vi "Main.vi"() -> ()   [LabVIEW 2019]
doc: "This template is for the Queued Message Handler design pattern.\n\nThe Event Handling Loop generates messages based on user interface actions.\n\nThe Message Handling Loop processes messages generated by the Event Handling Loop, or by other messages. The messages are string values, so new messages can be added easily to the Message Cases case structure in the Message Handling Loop. Each message cluster can also provide an optional value for Message Data, which is a variant that can be converted to whatever message-specific data is required."
uses:
  Type_Def/Onglet.ctl
  <vilib>/MakerHub/PS4-Controller/Private/Type Defs/Indicators/Controller.ctl
  <vilib>/MakerHub/PS4-Controller/Private/Type Defs/Indicators/Square.ctl
  <vilib>/MakerHub/PS4-Controller/Private/Type Defs/Indicators/X.ctl
  <vilib>/MakerHub/PS4-Controller/Private/Type Defs/Indicators/Circle.ctl
  <vilib>/MakerHub/PS4-Controller/Private/Type Defs/Indicators/Triangle.ctl
  <vilib>/MakerHub/PS4-Controller/Private/Type Defs/Indicators/L1.ctl
  <vilib>/MakerHub/PS4-Controller/Private/Type Defs/Indicators/R1.ctl
  <vilib>/MakerHub/PS4-Controller/Private/Type Defs/Indicators/Share.ctl
  <vilib>/MakerHub/PS4-Controller/Private/Type Defs/Indicators/Options.ctl
  <vilib>/MakerHub/PS4-Controller/Private/Type Defs/Indicators/PS.ctl
  <vilib>/MakerHub/PS4-Controller/Private/Type Defs/Indicators/Pad_Button.ctl
  <vilib>/MakerHub/PS4-Controller/Private/Type Defs/Indicators/Dpad.ctl
  <vilib>/MakerHub/PS4-Controller/Private/Type Defs/Indicators/Slider.ctl
  <vilib>/MakerHub/PS4-Controller/Private/Type Defs/Buttons.ctl
  <vilib>/MakerHub/PS4-Controller/Private/Type Defs/Axis.ctl
  <vilib>/MakerHub/PS4-Controller/Private/Type Defs/Indicators/DPad Enum.ctl
  Sous-Vi/SSH/SSH Library/Connection Info..cluster.ctl
  Sous-Vi/SSH/SSH Library/Password..cluster.ctl
  Sous-Vi/SSH/SSH Library/Private Public Key..cluster.ctl
  controls/UI Data.ctl
  Type_Def/Data.ctl
  Sous-Vi/SSH/SSH Library/connect_password.vi
  Sous-Vi/SSH/SSH Library/connect_key.vi
  support/Message Queue/Enqueue Message (Single).vi
  <vilib>/Utility/error.llb/Error Cluster From Error Code.vi
  <vilib>/Instr/_visa.llb/VISA Configure Serial Port (Instr).vi
  <vilib>/MakerHub/PS4-Controller/Public/Open First Controller.vi
  <vilib>/Utility/inputDevices.llb/closeJoystick.vi
  <vilib>/Utility/inputDevices.llb/joystickAcquire.vi
  Global/Global_1.vi
  <vilib>/ErrorRing/Error Ring.xnode
  support/Message Queue/Message Queue.lvlib
  support/User Event - Stop/User Event - Stop.lvlib
  <vilib>/MakerHub/PS4-Controller/LMH-PS4.lvlib
  Sous-Vi/SSH/SSH Library/LabSSH.lvlib
panel:
  out "OTHER 2":bool
  in  "Vitesse (ms)":u32(slide)=400 step=100 scale=600.0..100.0
  out "StatCom 2":bool
  in  "Putty":bool
  in  "Stop_Hexap":bool
  in  "Start_Hexap":bool
  in  "Stop COM":bool
  in  "Start COM":bool
  out "StatControll":bool
  out "StatCom":bool
  in  "Home Button":bool
  in  "Preferences Button":bool
  in  "Tab Control":T1
  in  "External_C":enum32{"PS4", "OTHER"}(tab)
  out "PS4 Controller":T2={"Square Button"=FALSE, "X Button"=FALSE, "Circle Button"=FALSE, "Triangle Button"=FALSE, "L1"=FALSE, "R1"=FALSE, "Share Button"=FALSE, "Options Button"=FALSE, "PS Button"=FALSE, "Pad Button"=FALSE, "D-Pad"=5, "L2"=0, "R2"=0, "Thumbstick_Left"={[], []}, "Thumbstick_Right"={[], []}} {"R2" scale=-32768.0..32767.0; "L2" scale=-32768.0..32767.0}
  out "PS4 Buttons":T15
  out "PS4 All Axis":T16
  out "axis info":T18
  out "button":T19
  out "direction info":T20
  out "Nuber of joysticks found:":i32
  in  "Joystick Number":i32
  out "Joystick in Use":T21={"axes total"=6, "buttons total"=14, "pov total"=1, "device name"="Wireless Controller"}
  out "Txt Display":string
  out "button 10":bool
  out "button 9":bool
  out "button 8":bool
  out "button 6":bool
  out "button 7":bool
  out "button 5":bool
  out "button 4":bool
  out "button 3":bool
  out "button 2":bool
  out "button 1":bool
  in  "Type External":enum16{"PS4 commander", "Other"}(ring)
  in  "Button 2":T22
  in  "Right joystick Horizontal 2":u8(slide) scale=3.0..253.0
  in  "Right  joystick Vertical 2":u8(slide) scale=3.0..253.0
  in  "Left joystick Horizontal 2":u8(slide) scale=3.0..253.0
  in  "Left joystick Vertical 2":u8(slide) scale=3.0..253.0
  out "Chaîne":string
  in  "TCP":T23={"port"=8888, "adresse"="", "timeout ms"=1000, "connection ID"=refnum}
  in  "Send":bool
  out "Array 2":u8[](array[numeric]) format="%x"
  out "Array":u8[](array[numeric]) format="%x"
  in  "R/W":bool
  in  "USB":T24={"COM"="", "baud rate (9600)"=34800, "data bits (8)"=8, "parity (0:none)"=enum."None", "stop bits (10: 1 bit)"=10, "flow control (0:none)"=0, "timeout (10sec)"=100} {"stop bits (10: 1 bit)" items=["1.0"=10, "1.5"=15, "2.0"=20]; "flow control (0:none)" items=["None", "XON/XOFF", "RTS/CTS", "XON/XOFF & RTS/CTS", "DTR/DSR", "XON/XOFF & DTR/DSR"]}
  in  "Send_L":bool
  in  "SSH_Connect":bool
  out "Method Response":string
  out "Connected":bool
  in  "Commande":string
  out "Output":string
  in  "Expected Response":string
  in  "Connection Type":enum16{"Password", "Private Key"}(ring)
  in  "Connection Name":string="ERAA_HEXAP"
  in  "Private_Public Key":T25
  in  "Password":T26={"Password"="edison"}
  in  "Connection Info.":T27={"Remote"="192.168.43.226", "Username"="root", "Port (22)"=22}
  out "error_":errorcluster
  out "Chaîne_CONTROLLER":string
  out "Chaîne_USB/WIFI":string
  out "error_Read_Com_SSH":errorcluster
  out "error_Send_Com_SSH":errorcluster
  out "Hexap_ON":bool
  out "Start/Stop COM":bool
  out "USB/WIFI":bool
  out "COM_OK":bool
  out "Init_Controller_OK":bool
  out "Init_COM_OK":bool
  out "Button":T22
  out "Right joystick Horizontal":u8(slide) scale=3.0..253.0
  out "Right  joystick Vertical":u8(slide) scale=3.0..253.0
  out "Left joystick Horizontal":u8(slide) scale=3.0..253.0
  out "Left joystick Vertical":u8(slide) scale=3.0..253.0
  out "Controller_OK":bool
  out "Tab_Ref":refnum<vi>[](array[refnum])
  out "error_OpenUSB":errorcluster
  out "CONTROLER":bool
  out "OTHER":bool
  out "error_Controller":errorcluster
  out "error_Send_Data":errorcluster
  out "error_OpenManette 2":errorcluster
  in  "Search Button":bool
  in  "Settings Button":bool
  in  "Type Comm":T28(ring)
  in  "Type Connexion":enum16{"Connexion USB", "Connexion WIFI"}(ring)=enum."Connexion WIFI"
  # "Debeugue SSH Selement en Exe"
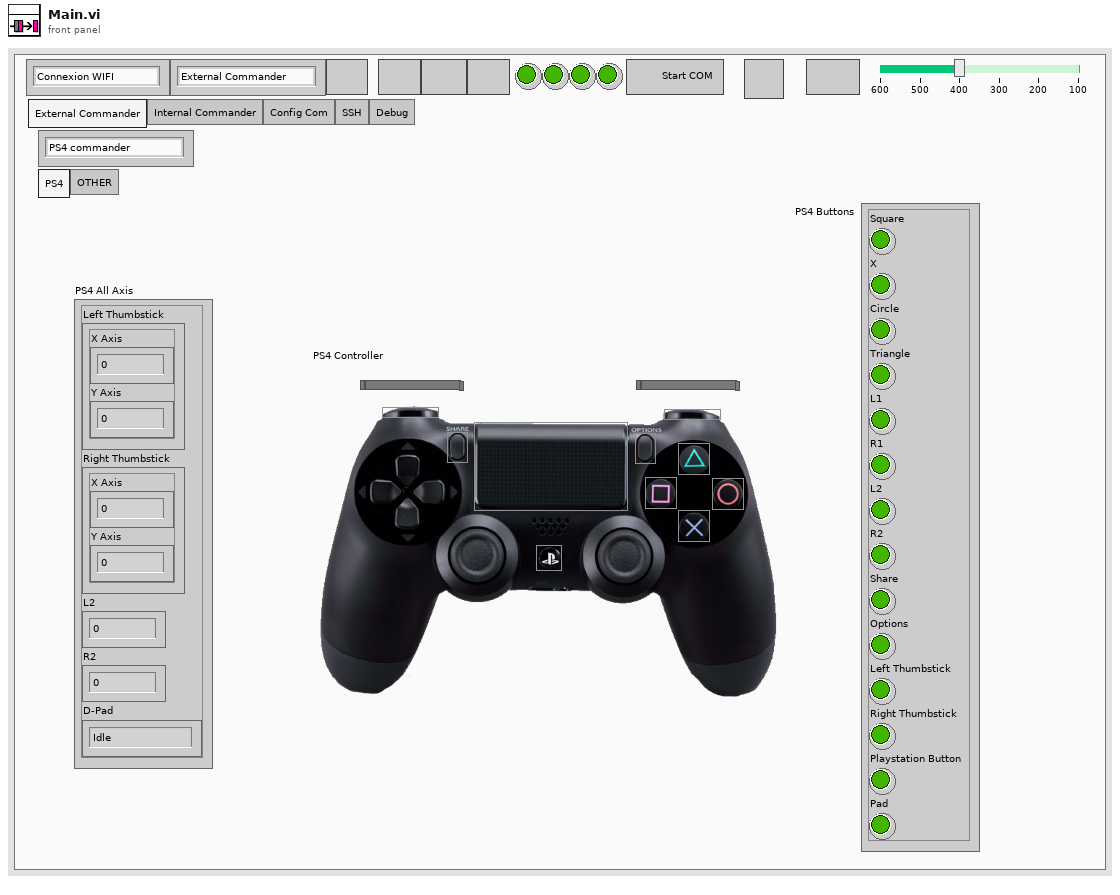
[diagram p1: front panel]
types:
  T1 = typedef "Onglet.ctl" = enum32{"External Commander", "Internal Commander", "Config Com", "SSH", "Debug"}
  T2 = typedef "LMH-PS4.lvlib/Controller.ctl" = cluster{"Square Button":T3, "X Button":T4, "Circle Button":T5, "Triangle Button":T6, "L1":T7, "R1":T8, "Share Button":T9, "Options Button":T10, "PS Button":T11, "Pad Button":T12, "D-Pad":T13, "L2":T14, "R2":T14, "Thumbstick_Left":cluster{i32[], i32[]}, "Thumbstick_Right":cluster{i32[], i32[]}}
  T3 = typedef "LMH-PS4.lvlib/Square.ctl" = bool
  T4 = typedef "LMH-PS4.lvlib/X.ctl" = bool
  T5 = typedef "LMH-PS4.lvlib/Circle.ctl" = bool
  T6 = typedef "LMH-PS4.lvlib/Triangle.ctl" = bool
  T7 = typedef "LMH-PS4.lvlib/L1.ctl" = bool
  T8 = typedef "LMH-PS4.lvlib/R1.ctl" = bool
  T9 = typedef "LMH-PS4.lvlib/Share.ctl" = bool
  T10 = typedef "LMH-PS4.lvlib/Options.ctl" = bool
  T11 = typedef "LMH-PS4.lvlib/PS.ctl" = bool
  T12 = typedef "LMH-PS4.lvlib/Pad_Button.ctl" = bool
  T13 = typedef "LMH-PS4.lvlib/Dpad.ctl" = u16
  T14 = typedef "LMH-PS4.lvlib/Slider.ctl" = i32
  T15 = typedef "LMH-PS4.lvlib/Buttons.ctl" = cluster{"Square":bool, "X":bool, "Circle":bool, "Triangle":bool, "L1":bool, "R1":bool, "L2":bool, "R2":bool, "Share":bool, "Options":bool, "Left Thumbstick":bool, "Right Thumbstick":bool, "Playstation Button":bool, "Pad":bool}
  T16 = typedef "LMH-PS4.lvlib/Axis.ctl" = cluster{"Left Thumbstick":cluster{"X Axis":i32, "Y Axis":i32}, "Right Thumbstick":cluster{"X Axis":i32, "Y Axis":i32}, "L2":i32, "R2":i32, "D-Pad":T17}
  T17 = typedef "LMH-PS4.lvlib/DPad Enum.ctl" = enum16{"Idle", "Up", "Up / Right", "Right", "Down / Right", "Down", "Down / Left", "Left", "Up / Left"}
  T18 = cluster{"X axis":i32, "Y axis":i32, "Z axis":i32, "X axis rotation":i32, "Y axis rotation":i32, "Z axis rotation":i32, "U axis":i32, "V axis":i32}
  T19 = cluster{"button[1]":bool, "button[2]":bool, "button[3]":bool, "button[4]":bool, "button[5]":bool, "button[6]":bool, "button[7]":bool, "button[8]":bool, "button[9]":bool, "button[10]":bool}
  T20 = cluster{"pov 1":i32, "pov 2":i32, "pov 3":i32, "pov 4":i32}
  T21 = cluster{"axes total":u32, "buttons total":u32, "pov total":u32, "device name":string}
  T22 = cluster{"R1":bool, "R2":bool, "R3":bool, "L4":bool, "L5":bool, "L6":bool, "LT":bool, "RT":bool}
  T23 = cluster{"port":u16, "adresse":string, "timeout ms":i32, "connection ID":refnum<k5>}
  T24 = cluster{"COM":refnum<visa-resource-name>, "baud rate (9600)":u32, "data bits (8)":u16, "parity (0:none)":enum16{"None", "Odd", "Even", "Mark", "Space"}, "stop bits (10: 1 bit)":u16, "flow control (0:none)":u16, "timeout (10sec)":u32}
  T25 = typedef "LabSSH.lvlib/Private Public Key..cluster.ctl" = cluster{"Private Key":path, "Passphrase":string}
  T26 = typedef "LabSSH.lvlib/Password..cluster.ctl" = cluster{"Password":string}
  T27 = typedef "LabSSH.lvlib/Connection Info..cluster.ctl" = cluster{"Remote":string, "Username":string, "Port (22)":i32}
  T28 = enum16{"External Commander", "Internal Commander"}
  T29 = typedef "UI Data.ctl" = cluster{"Boolean <Replace Me>":bool, "String <Replace Me>":string, "Numeric <Replace Me>":dbl, "Do Something Ref":refnum<vi>, "Do Something Else Ref":refnum<vi>, "Data Display Ref":refnum<vi>, "Exit Button Ref":refnum<vi>}
  T30 = typedef "Message Queue.lvlib/All Message Queues.ctl" = cluster{"UI":refnum<queue>, "UI 2":refnum<queue>, "UI 3":refnum<queue>, "UI 4":refnum<queue>}
  T31 = typedef "Data.ctl" = cluster{"Data":string, "COM":refnum<visa-resource-name>}
  T32 = typedef "LMH-PS4.lvlib/PS4 Controller Ref.ctl" = cluster{"Controller Ref":refnum<k1>, "PS4 Events Ref":refnum<event-registration>, "Worker Ref":refnum<vi>}
  T33 = cluster{"axes total":u32, "buttons total":u32, "pov total":u32, "device name":string}[]
  T34 = cluster{"button 1":bool, "button 2":bool, "button 3":bool, "button 4":bool, "button 5":bool, "button 6":bool, "button 7":bool, "button 8":bool, "button 9":bool, "button 10":bool, "button 11":bool, "button 12":bool, "button 13":bool, "button 14":bool, "button 15":bool, "button 16":bool, "button 17":bool, "button 18":bool, "button 19":bool, "button 20":bool, "button 21":bool, "button 22":bool, "button 23":bool, "button 24":bool, "button 25":bool, "button 26":bool, "button 27":bool, "button 28":bool, "button 29":bool, "button 30":bool, "button 31":bool, "button 32":bool}
  T35 = cluster{"button info[0]":bool, "button info[1]":bool, "button info[2]":bool, "button info[3]":bool, "button info[4]":bool, "button info[5]":bool, "button info[6]":bool, "button info[7]":bool, "button info[8]":bool, "button info[9]":bool}
  T36 = cluster{"Boolean array[0]":bool, "Boolean array[1]":bool, "Boolean array[2]":bool, "Boolean array[3]":bool, "Boolean array[4]":bool, "Boolean array[5]":bool, "Boolean array[6]":bool, "Boolean array[7]":bool, "Boolean array[8]":bool}
  T37 = enum32{"External Commander", "Internal Commander", "Config Com", "SSH", "Debug"}
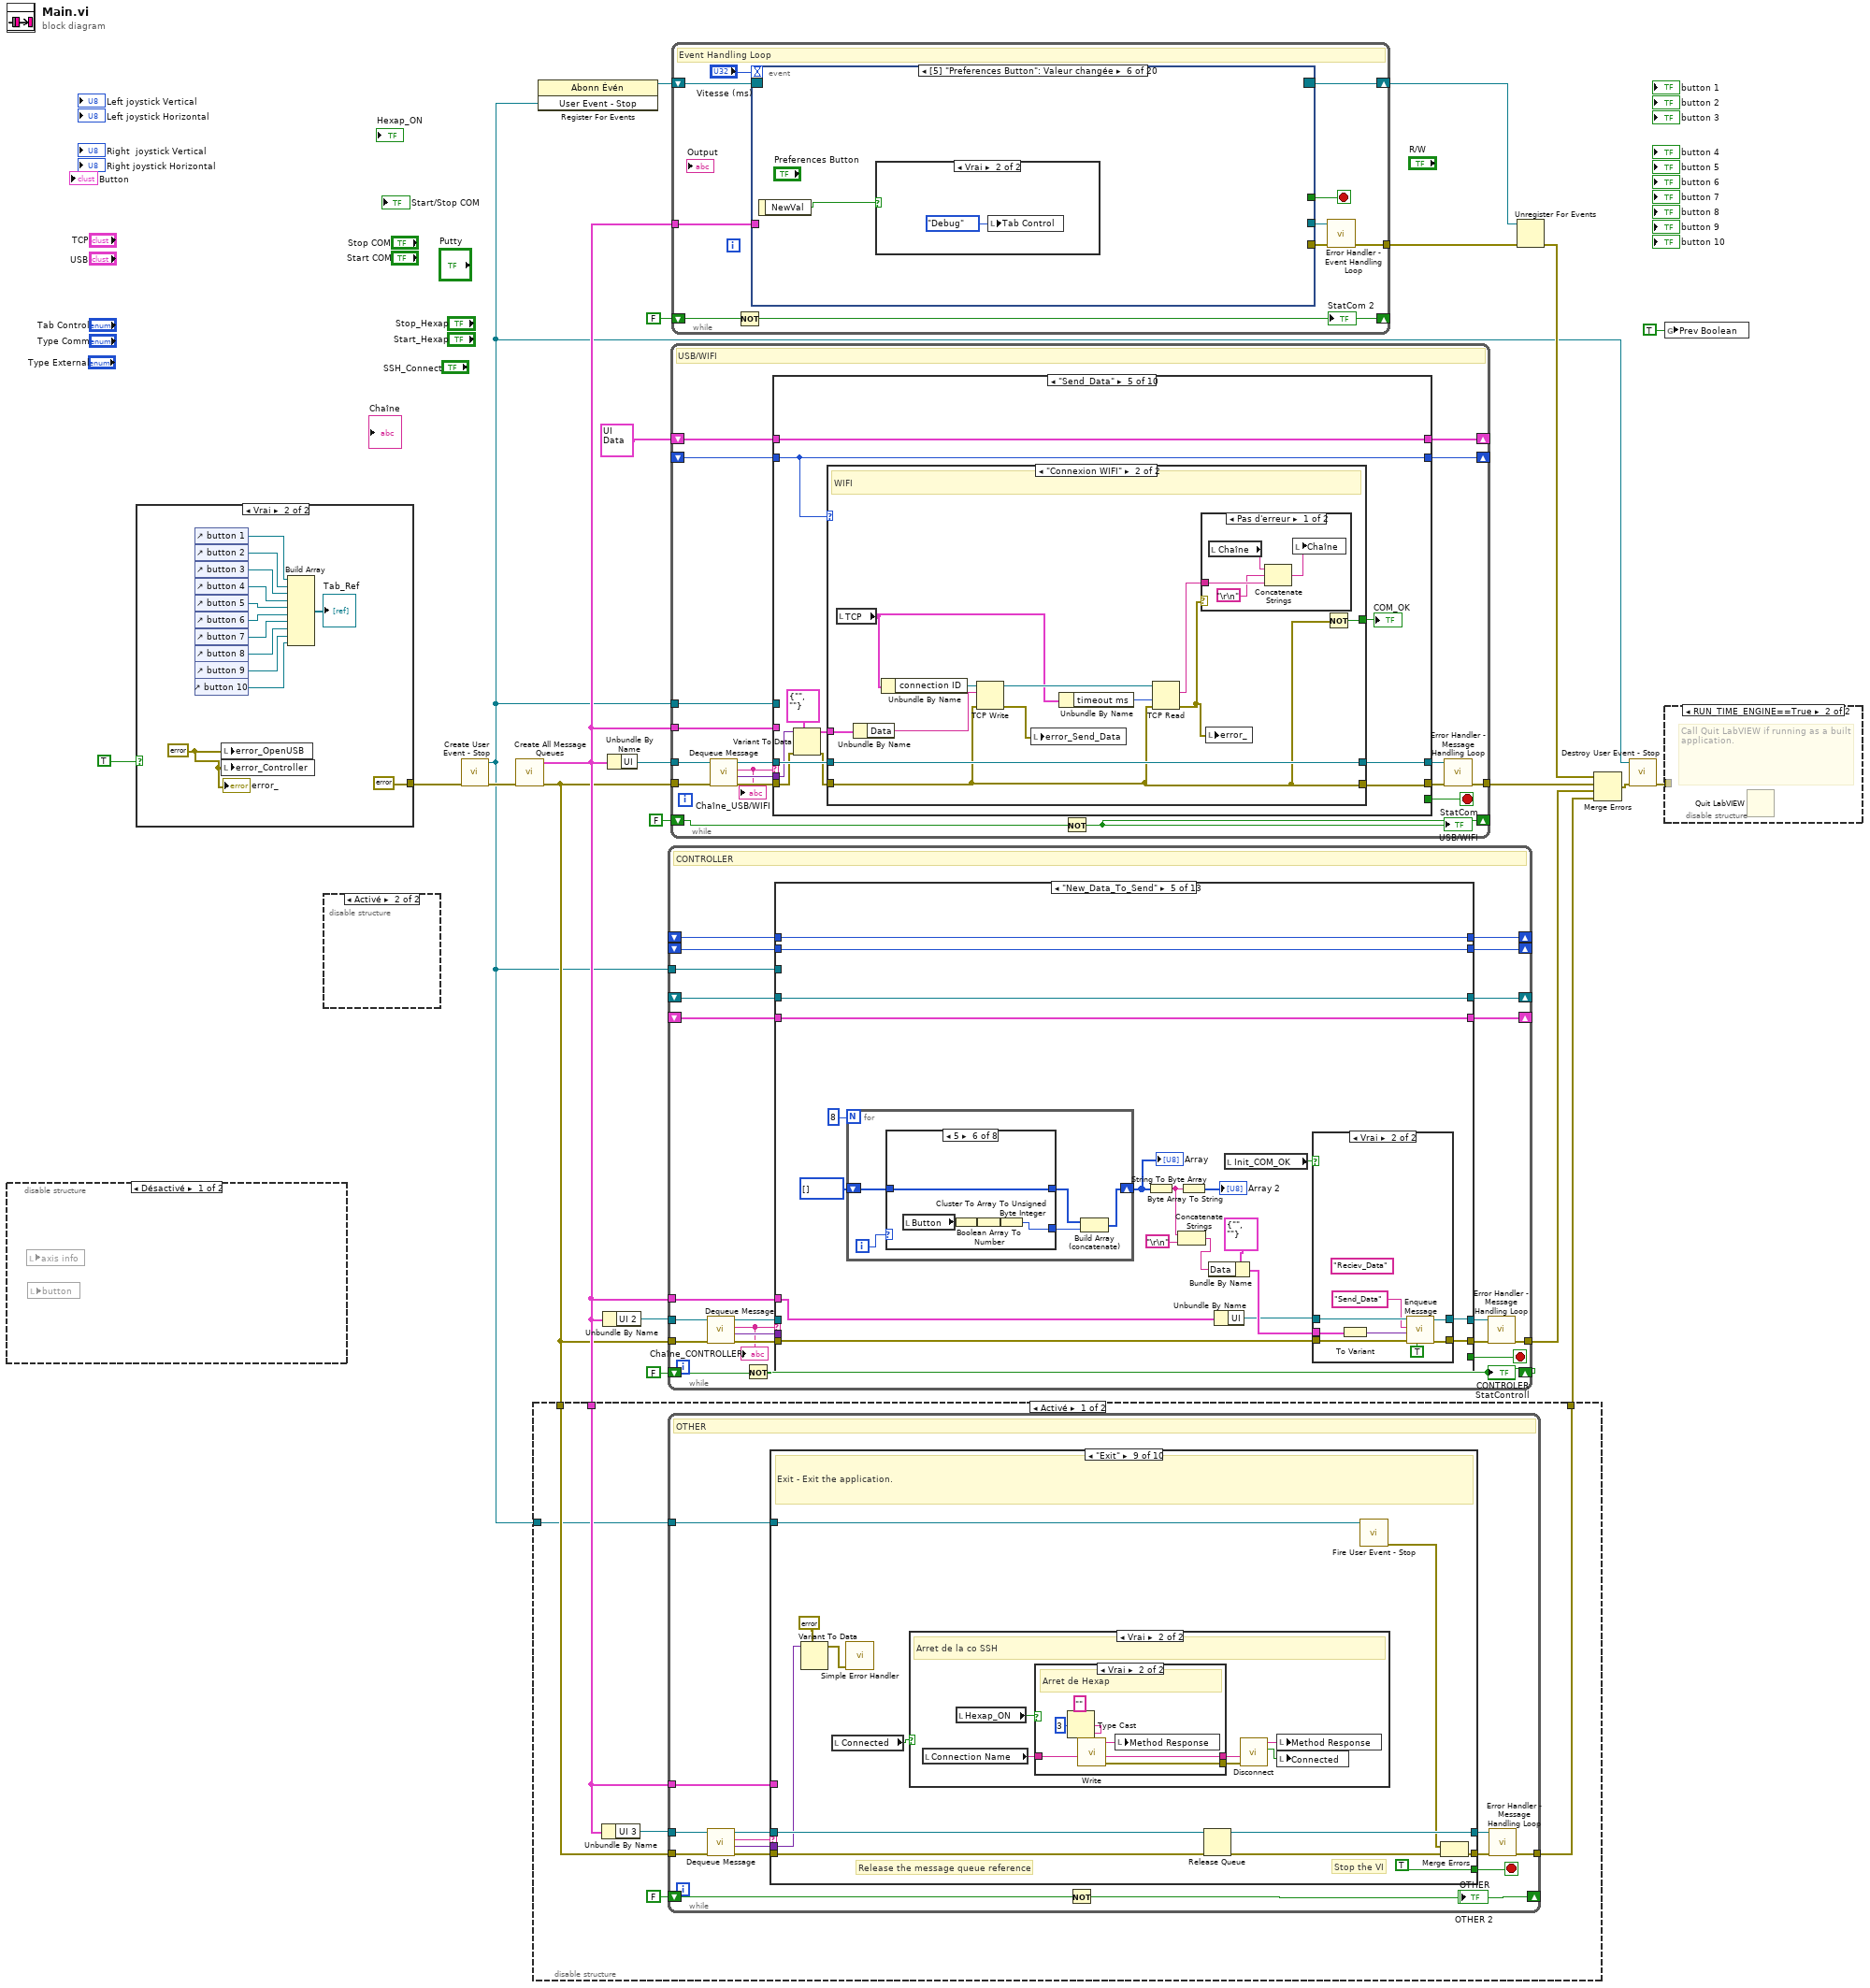
[diagram p0: block diagram]
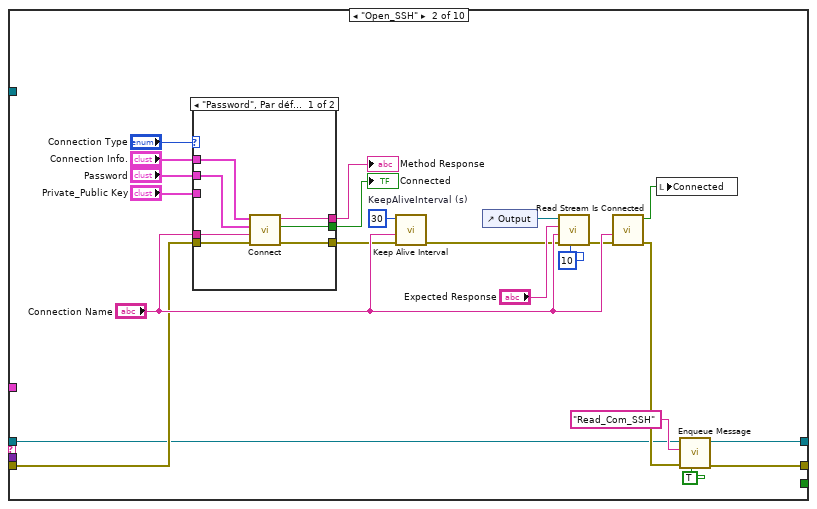
[diagram p4: hidden frame]
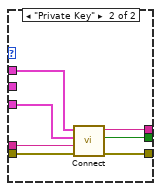
[diagram p5: hidden frame]
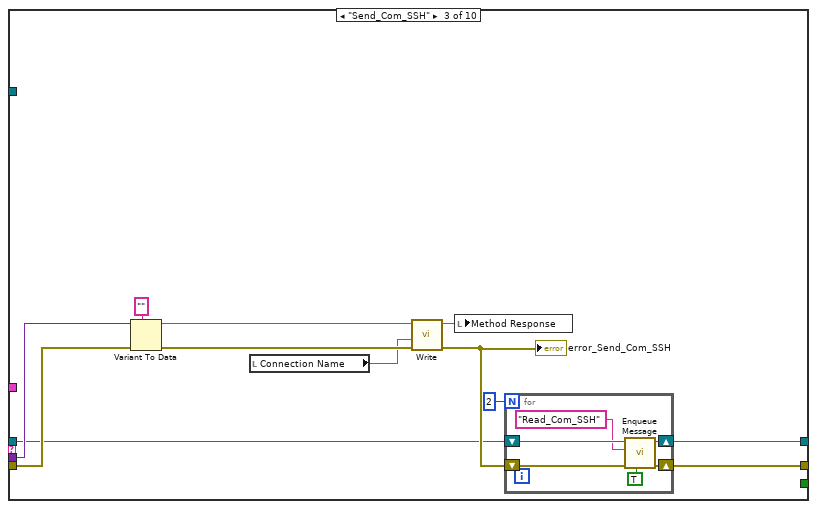
[diagram p6: hidden frame]
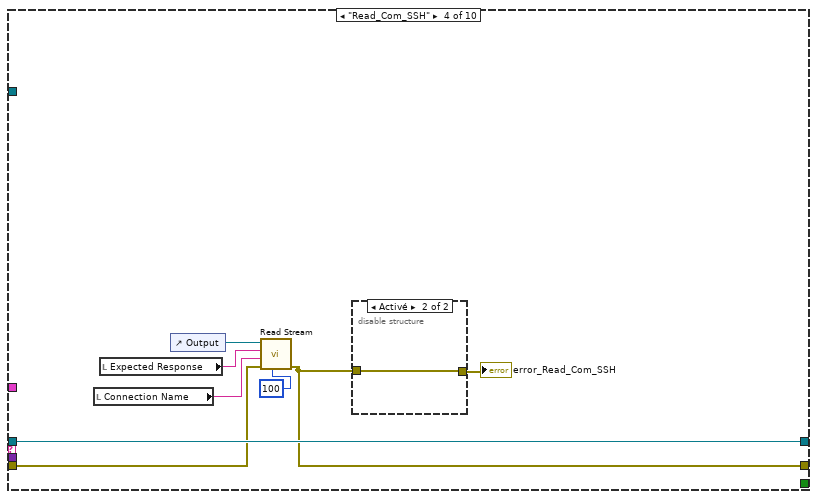
[diagram p7: hidden frame]
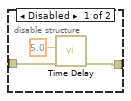
[diagram p8: hidden frame]
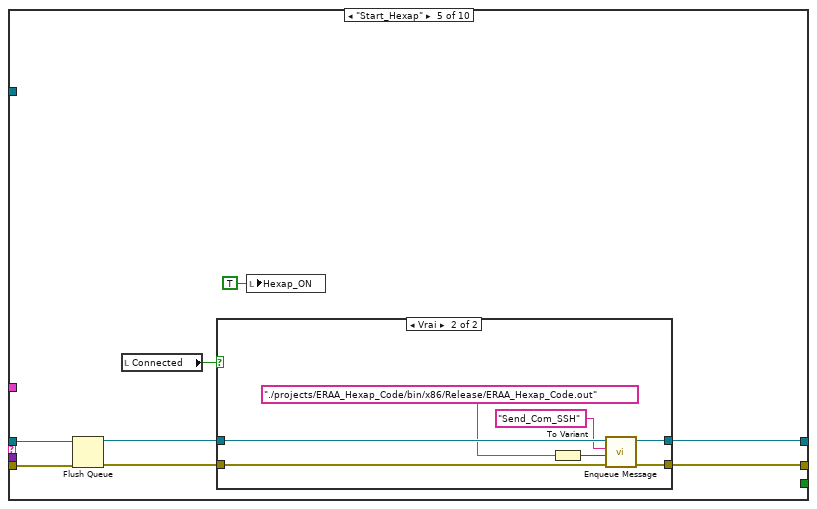
[diagram p9: hidden frame]
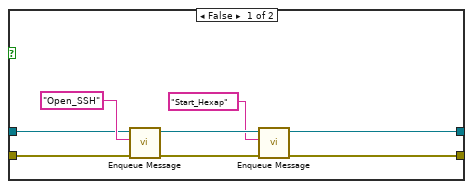
[diagram p10: hidden frame]
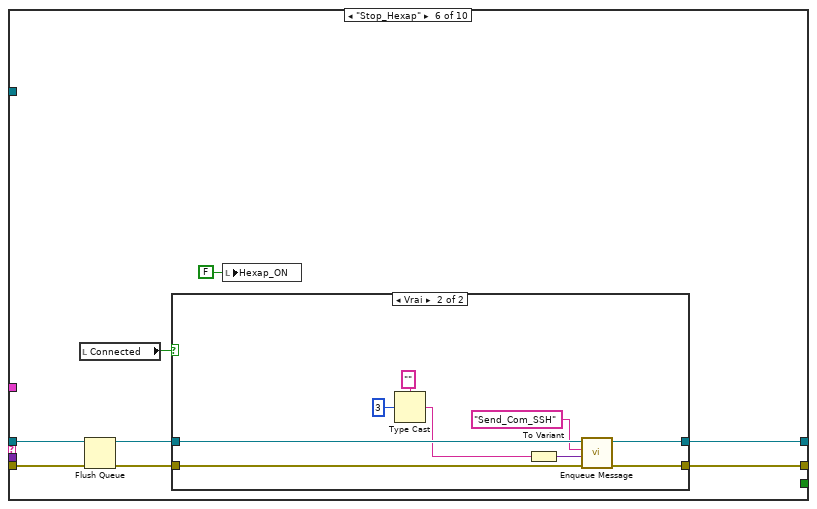
[diagram p11: hidden frame]
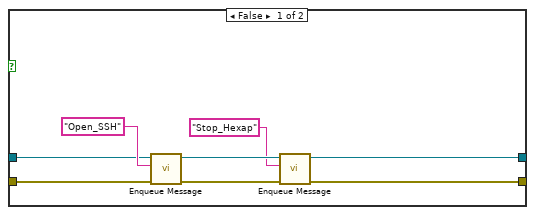
[diagram p12: hidden frame]
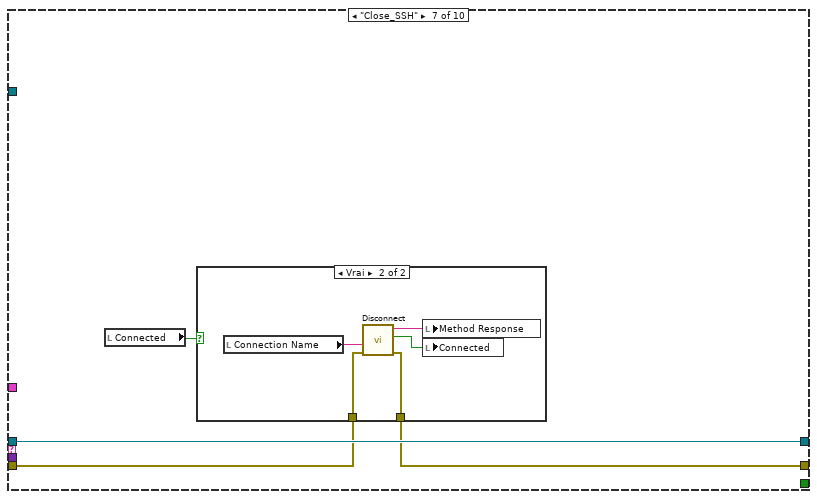
[diagram p13: hidden frame]
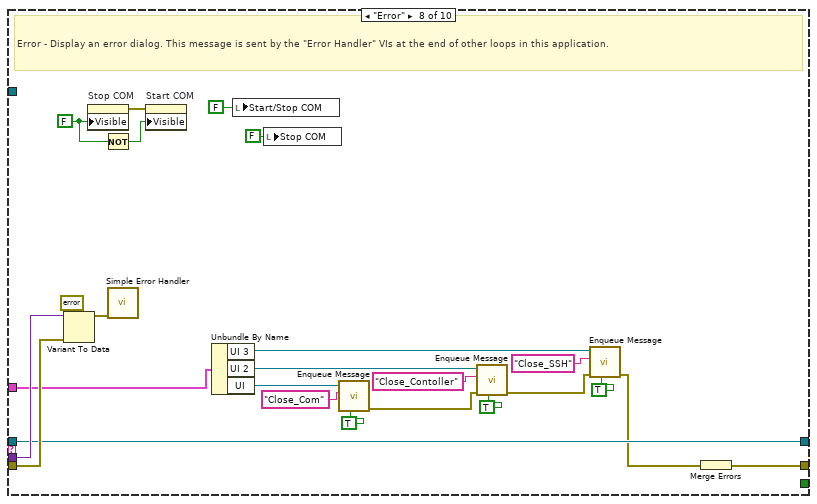
[diagram p15: hidden frame]
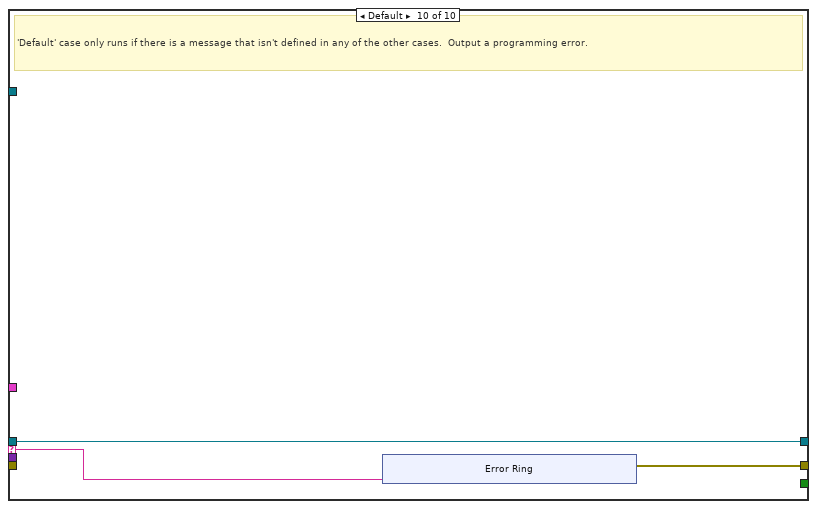
[diagram p18: hidden frame]
diagram:
  n1 = disable-structure shown="Désactivé" {
    frame Disabled {
      n2 = local read "axis info"() -> ()  [unwired: 1 in]
      n3 = local read "button"() -> ()  [unwired: 1 in]
    }
    frame Enabled {
    }
  }
  n4 = case shown="Vrai" TRUE {
    tunnel: [_ errorcluster {"status"=FALSE, "code"=0, "source"=""} ("error out")] -> w7
    frame False {
    }
    frame True {
      w23 = errorcluster {"status"=FALSE, "code"=0, "source"=""} ("error out")
      n5 = control-ref of="button 1"() -> (w25:refnum<vi>)
      n6 = control-ref of="button 2"() -> (w26:refnum<vi>)
      n7 = control-ref of="button 3"() -> (w27:refnum<vi>)
      n8 = control-ref of="button 4"() -> (w28:refnum<vi>)
      n9 = control-ref of="button 5"() -> (w29:refnum<vi>)
      n10 = control-ref of="button 6"() -> (w30:refnum<vi>)
      n11 = control-ref of="button 7"() -> (w31:refnum<vi>)
      n12 = control-ref of="button 8"() -> (w32:refnum<vi>)
      n13 = control-ref of="button 9"() -> (w33:refnum<vi>)
      n14 = control-ref of="button 10"() -> (w34:refnum<vi>)
      n15 = local write "error_OpenUSB"(w23) -> ()
      n16 = local write "error_Controller"(w23) -> ()
      n17 = Build Array(w25, w26, w27, w28, w29, w30, w31, w32, w33, w34) -> (→"Tab_Ref":refnum<vi>[])
      "error_" <- w23
    }
  }
  n18 = disable-structure shown="Activé" {
    frame Disabled {
      n19 = call <vilib>:"Disconnect Network Resource.vi"() -> ()  [unwired: 7 in, 1 out]
      n20 = call <vilib>:"Add Network Resource.vi"() -> ()  [unwired: 7 in, 1 out]
      n21 = global read "Global_1.vi" item#-1() -> ()  [unwired: 1 in]
    }
    frame Enabled {
    }
  }
  n22 = call "Create User Event - Stop.vi"("error in (no error)"=w7) -> ("error out"=w20:errorcluster, "User Event - Stop"=w1:refnum<user-event>)  [unwired: 9 in]
  n23 = call "Create All Message Queues.vi"("error in (no error)"=w20) -> ("error out"=w4:errorcluster, "Message Queues out"=w10:T30)  [unwired: 9 in]
  n24 = disable-structure shown="Activé" {
    disable-tunnel: w10 -> [w37 _]
    disable-tunnel: [w40 w240] -> w9
    disable-tunnel: w4 -> [w38 w240]
    disable-tunnel: w1 -> [w36 _]
    frame Enabled {
      n25 = Unbundle By Name(w37) -> ("UI 3"=w41:refnum<queue>)
      n26 = while {
        tunnel: w41 -> [w51]
        shift-right: [w42] -> _
        shift-left: FALSE -> [w46]
        tunnel: w38 -> [w45]
        tunnel: [w49] -> w40
        tunnel: w37 -> [w44]
        tunnel: w36 -> [w43]
        stop <- w55 stop-if-true
        # "OTHER"
        n27 = call "Dequeue Message.vi"("error in (no error)"=w45, "Message Queue"=w51) -> ("error out"=w54:errorcluster, "Message Data"=w52:variant, "Message"=w53:string, "dup Message Queue"=w50:refnum<queue>)  [unwired: 6 in]
        n28 = case "Message Cases" shown="\"Exit\"" w53 {
          selector: w53 -> [_ _ _ _ _ _ _ _ _ w231]
          tunnel: w50 -> [w57 w60 w96 w119 w127 w148 w175 w200 w216 w230]
          tunnel: w54 -> [w56 w61 w97 w113 w126 w147 w173 w205 w212 _]
          tunnel: [w56 w58 w94 w112 w124 w149 w172 w201 w213 w232] -> w48
          tunnel: [_ _ _ _ _ _ _ _ TRUE _] -> w55
          tunnel: w52 -> [_ _ w98 _ _ _ _ w204 w209 _]
          tunnel: [w57 w59 w95 w119 w125 w150 w175 w200 w216 w230] -> w47
          tunnel: w44 -> [_ _ _ _ _ _ _ w188 _ _]
          tunnel: w43 -> [_ _ _ _ _ _ _ _ w206 _]
          frame "Initialize" {
            # "Initialize - All initialization work should take place in this message, since other loops can potentially enqueue messages that execute immediately after this one."
          }
          frame "Open_SSH" {
            w62 = 30  # KeepAliveInterval (s)
            n29 = case shown="\"Password\", Par défaut" "Connection Type" {
              tunnel: "Connection Info." -> [w86 w91]
              tunnel: "Password" -> [w85 _]
              tunnel: "Private_Public Key" -> [_ w90]
              tunnel: w61 -> [w84 w93]
              tunnel: [w83 w92] -> w72
              tunnel: "Connection Name" -> [w82 w89]
              tunnel: [w81 w88] -> w71
              tunnel: [w80 w87] -> w70
              frame "Password", Default {
                n30 = call-poly "Connect.vi"("error in (no error)"=w84, "Connection Name"=w82, "Password"=w85, "Connection Info."=w86) -> ("error out"=w83:errorcluster, "isSshConnected"=w80:bool, "Return String"=w81:string)  [unwired: 5 in]
              }
              frame "Private Key" {
                n31 = call-poly "Connect.vi"("error in (no error)"=w93, "Connection Name"=w89, "Private_Public Key"=w90, "Connection Info."=w91) -> ("error out"=w92:errorcluster, "isSshConnected"=w87:bool, "Return String"=w88:string)  [unwired: 5 in]
              }
            }
            "Connected" <- w70
            "Method Response" <- w71
            n32 = call "Keep Alive Interval.vi"("error in (no error)"=w72, "Connection Name"="Connection Name", "KeepAliveInterval (s)"=w62) -> ("error out"=w74:errorcluster)  [unwired: 8 in]
            n33 = control-ref of="Output"() -> (w73:refnum<vi>)
            n34 = call "Read Stream.vi"("Timout (ms)"=10 ("Timout (s)"), "error in (no error)"=w74, "Connection Name"="Connection Name", "Expected Response"="Expected Response", "Output ref"=w73) -> ("error out"=w76:errorcluster)  [unwired: 6 in]
            n35 = call "Is Connected.vi"("error in (no error)"=w76, "Connection Name"="Connection Name") -> ("error out"=w79:errorcluster, "isSshConnected"=w78:bool)  [unwired: 8 in]
            n36 = local write "Connected"(w78) -> ()
            n37 = call-poly "Enqueue Message.vi"("Priority Message? (F)"=TRUE, "error in (no error)"=w79, "Message"="Read_Com_SSH", "Message Queue"=w60) -> ("error out"=w58:errorcluster, "dup Message Queue"=w59:refnum<queue>)  [unwired: 6 in]
          }
          frame "Send_Com_SSH" {
            n38 = Variant To Data(error in=w97, type="" ("Commande"), Variant=w98) -> (data=w104:string, error out=w102:errorcluster)
            n39 = local read "Connection Name"() -> (w101:string)
            n40 = call "Write.vi"("error in (no error)"=w102, "Connection Name"=w101, "Command"=w104) -> ("error out"=w99:errorcluster, "Return String"=w103:string)  [unwired: 7 in]
            "error_Send_Com_SSH" <- w99
            n41 = local write "Method Response"(w103) -> ()
            n42 = for {
              N: 2 -> [_]
              shift-right: [w109] -> w95
              shift-left: w96 -> [w110]
              shift-right: [w111] -> w94
              shift-left: w99 -> [w107]
              n43 = call-poly "Enqueue Message.vi"("Priority Message? (F)"=TRUE, "error in (no error)"=w107, "Message"="Read_Com_SSH", "Message Queue"=w110) -> ("error out"=w111:errorcluster, "dup Message Queue"=w109:refnum<queue>)  [unwired: 6 in]
            }
          }
          frame "Read_Com_SSH" {
            n44 = local read "Connection Name"() -> (w117:string)
            n45 = local read "Expected Response"() -> (w116:string)
            n46 = control-ref of="Output"() -> (w115:refnum<vi>)
            n47 = call "Read Stream.vi"("Timout (ms)"=100 ("Timout (s)"), "error in (no error)"=w113, "Connection Name"=w117, "Expected Response"=w116, "Output ref"=w115) -> ("error out"=w112:errorcluster)  [unwired: 6 in]
            n48 = disable-structure shown="Activé" {
              disable-tunnel: w112 -> [w121 w123]
              disable-tunnel: [w120 w123] -> w118
              frame Disabled {
                n49 = call "Time Delay"("error in (no error)"=w121, "Delay Time (s)"=5.0) -> ("error out"=w120:errorcluster)  [unwired: 9 in]
              }
              frame Enabled {
              }
            }
            "error_Read_Com_SSH" <- w118
          }
          frame "Start_Hexap" {
            n50 = Flush Queue(queue=w127, error in (no error)=w126) -> (queue out=w130:refnum<queue>, error out=w131:errorcluster)  [unwired: 1 out]
            n51 = local read "Connected"() -> (w129:bool)
            n52 = case shown="Vrai" w129 {
              tunnel: w130 -> [w138 w146]
              tunnel: w131 -> [w137 w145]
              tunnel: [w134 w141] -> w125
              tunnel: [w133 w140] -> w124
              frame False {
                n53 = call-poly "Enqueue Message.vi"("error in (no error)"=w137, "Message"="Open_SSH", "Message Queue"=w138) -> ("error out"=w135:errorcluster, "dup Message Queue"=w136:refnum<queue>)  [unwired: 7 in]
                n54 = call-poly "Enqueue Message.vi"("error in (no error)"=w135, "Message"="Start_Hexap", "Message Queue"=w136) -> ("error out"=w133:errorcluster, "dup Message Queue"=w134:refnum<queue>)  [unwired: 7 in]
              }
              frame True {
                n55 = To Variant(anything="./projects/ERAA_Hexap_Code/bin/x86/Release/ERAA_Hexap_Code.out" ("Message")) -> (Variant=w143:variant)
                n56 = call-poly "Enqueue Message.vi"("error in (no error)"=w145, "Message Data"=w143, "Message"="Send_Com_SSH", "Message Queue"=w146) -> ("error out"=w140:errorcluster, "dup Message Queue"=w141:refnum<queue>)  [unwired: 6 in]
              }
            }
            n57 = local write "Hexap_ON"(TRUE ("Hexap_ON")) -> ()
          }
          frame "Stop_Hexap" {
            n58 = local read "Connected"() -> (w152:bool)
            n59 = Flush Queue(queue=w148, error in (no error)=w147) -> (queue out=w153:refnum<queue>, error out=w154:errorcluster)  [unwired: 1 out]
            n60 = case shown="Vrai" w152 {
              tunnel: w153 -> [w161 w171]
              tunnel: w154 -> [w160 w170]
              tunnel: [w157 w167] -> w150
              tunnel: [w156 w166] -> w149
              frame False {
                n61 = call-poly "Enqueue Message.vi"("error in (no error)"=w160, "Message"="Open_SSH", "Message Queue"=w161) -> ("error out"=w158:errorcluster, "dup Message Queue"=w159:refnum<queue>)  [unwired: 7 in]
                n62 = call-poly "Enqueue Message.vi"("error in (no error)"=w158, "Message"="Stop_Hexap", "Message Queue"=w159) -> ("error out"=w156:errorcluster, "dup Message Queue"=w157:refnum<queue>)  [unwired: 7 in]
              }
              frame True {
                n63 = Type Cast(type="", x=u8 3) -> (*(type *) &x=w163:string)
                n64 = To Variant(anything=w163) -> (Variant=w168:variant)
                n65 = call-poly "Enqueue Message.vi"("error in (no error)"=w170, "Message Data"=w168, "Message"="Send_Com_SSH", "Message Queue"=w171) -> ("error out"=w166:errorcluster, "dup Message Queue"=w167:refnum<queue>)  [unwired: 6 in]
              }
            }
            n66 = local write "Hexap_ON"(FALSE ("Hexap_ON")) -> ()
          }
          frame "Close_SSH" {
            n67 = local read "Connected"() -> (w174:bool)
            n68 = case shown="Vrai" w174 {
              tunnel: w173 -> [w176 w178]
              tunnel: [w176 w177] -> w172
              frame False {
              }
              frame True {
                n69 = local read "Connection Name"() -> (w181:string)
                n70 = call "Disconnect.vi"("error in (no error)"=w178, "Connection Name"=w181) -> ("error out"=w177:errorcluster, "isSshConnected"=w179:bool, "Return String"=w180:string)  [unwired: 7 in]
                n71 = local write "Method Response"(w180) -> ()
                n72 = local write "Connected"(w179) -> ()
              }
            }
          }
          frame "Error" {
            w186 = FALSE
            # "Error - Display an error dialog. This message is sent by the \"Error Handler\" VIs at the end of other loops in this application."
            n73 = Variant To Data(error in=w205, type=errorcluster {"status"=FALSE, "code"=0, "source"=""} ("error constant"), Variant=w204) -> (data=w202:errorcluster)  [unwired: 1 out]
            n74 = property on="Stop COM" class="Bool (strict)"("Visible"=w186) -> (error out=w184:errorcluster)  [unwired: 2 in, 1 out]
            n75 = Not(x=w186) -> (.not. x?=w185:bool)
            n76 = call <vilib>:"Simple Error Handler.vi"("error in (no error)"=w202) -> ()  [unwired: 4 in, 5 out]
            n77 = property on="Start COM" class="Bool (strict)"(error in=w184, "Visible"=w185) -> ()  [unwired: 1 in, 2 out]
            n78 = Unbundle By Name(w188) -> ("UI 3"=w190:refnum<queue>, "UI 2"=w194:refnum<queue>, "UI"=w197:refnum<queue>)
            n79 = local write "Start/Stop COM"(FALSE ("Start/Stop COM")) -> ()
            n80 = local write "Stop COM"(FALSE ("Stop COM")) -> ()
            n81 = call-poly "Enqueue Message.vi"("Priority Message? (F)"=TRUE, "Message"="Close_Com", "Message Queue"=w197) -> ("error out"=w193:errorcluster)  [unwired: 7 in, 1 out]
            n82 = call-poly "Enqueue Message.vi"("Priority Message? (F)"=TRUE, "error in (no error)"=w193, "Message"="Close_Contoller", "Message Queue"=w194) -> ("error out"=w189:errorcluster)  [unwired: 6 in, 1 out]
            n83 = call-poly "Enqueue Message.vi"("Priority Message? (F)"=TRUE, "error in (no error)"=w189, "Message"="Close_SSH", "Message Queue"=w190) -> ("error out"=w187:errorcluster)  [unwired: 6 in, 1 out]
            n84 = Merge Errors(w187) -> (w201:errorcluster)
          }
          frame "Exit" {
            # "Stop the VI"
            # "Release the message queue reference"
            # "Exit - Exit the application."
            n85 = Variant To Data(type=errorcluster {"status"=FALSE, "code"=0, "source"=""} ("error constant"), Variant=w209) -> (data=w210:errorcluster)  [unwired: 1 in, 1 out]
            n86 = local read "Connected"() -> (w208:bool)
            n87 = call <vilib>:"Simple Error Handler.vi"("error in (no error)"=w210) -> ()  [unwired: 4 in, 5 out]
            n88 = case shown="Vrai" w208 {
              frame False {
              }
              frame True {
                # "Arret de la co SSH"
                n89 = local read "Connection Name"() -> (w219:string)
                n90 = local read "Hexap_ON"() -> (w220:bool)
                n91 = case shown="Vrai" w220 {
                  tunnel: w219 -> [w223 w229]
                  tunnel: [w223 w229] -> w218
                  tunnel: [_ w228] -> w217
                  frame False {
                  }
                  frame True {
                    # "Arret de Hexap"
                    n92 = Type Cast(type="", x=u8 3) -> (*(type *) &x=w224:string)
                    n93 = call "Write.vi"("Connection Name"=w229, "Command"=w224) -> ("error out"=w228:errorcluster, "Return String"=w227:string)  [unwired: 8 in]
                    n94 = local write "Method Response"(w227) -> ()
                  }
                }
                n95 = call "Disconnect.vi"("error in (no error)"=w217, "Connection Name"=w218) -> ("isSshConnected"=w221:bool, "Return String"=w222:string)  [unwired: 7 in, 1 out]
                n96 = local write "Method Response"(w222) -> ()
                n97 = local write "Connected"(w221) -> ()
              }
            }
            n98 = Release Queue(queue=w216, error in (no error)=w212) -> (error out=w214:errorcluster)  [unwired: 1 in, 2 out]
            n99 = call "Fire User Event - Stop.vi"("User Event - Stop"=w206) -> ("error out"=w207:errorcluster)  [unwired: 10 in]
            n100 = Merge Errors(w207, w214) -> (w213:errorcluster)
          }
          frame Default {
            # "'Default' case only runs if there is a message that isn't defined in any of the other cases.  Output a programming error."
            n101 = xnode "Error Ring"("paramètre 0"=w231) -> ("sortie d'erreur"=w232:errorcluster)
          }
        }
        n102 = Not(x=w46) -> (.not. x?=w42:bool)
        "OTHER" <- w42
        "OTHER 2" <- w42
        n103 = call "Error Handler - Message Handling Loop.vi"("error in (no error)"=w48, "Message Queue"=w47) -> ("dup error in"=w49:errorcluster)  [unwired: 8 in, 1 out]
      }
    }
    frame Disabled {
    }
  }
  n104 = register-events(w1) -> (reference out=w13:refnum<event-registration>)  [unwired: 2 in, 1 out]
  n105 = Unbundle By Name(w10) -> ("UI 2"=w12:refnum<queue>)
  n106 = Unbundle By Name(w10) -> ("UI"=w21:refnum<queue>)
  n107 = while {
    tunnel: w12 -> [w258]
    tunnel: w4 -> [w261]
    tunnel: [w256] -> w11
    tunnel: w10 -> [w254]
    shift-right: [w252] -> _
    shift-left: _ -> [w251]
    shift-right: [w250] -> _
    shift-left: _ -> [w249]
    shift-right: [w248] -> _
    shift-left: _ -> [w247]
    shift-right: [w246] -> _
    shift-left: _ -> [w245]
    shift-right: [w243] -> _
    shift-left: FALSE -> [w244]
    tunnel: w1 -> [w242]
    stop <- w262 stop-if-true
    # "CONTROLLER"
    n108 = call "Dequeue Message.vi"("error in (no error)"=w261, "Message Queue"=w258) -> ("error out"=w260:errorcluster, "Message Data"=w259:variant, "Message"=w241:string, "dup Message Queue"=w257:refnum<queue>)  [unwired: 6 in]
    "Chaîne_CONTROLLER" <- w241
    n109 = Not(x=w244) -> (.not. x?=w243:bool)
    "CONTROLER" <- w243
    "StatControll" <- w243
    n110 = case "Message Cases" shown="\"New_Data_To_Send\"" w241 {
      selector: w241 -> [_ _ _ _ _ _ _ _ _ _ _ _ w644]
      tunnel: w257 -> [w266 w285 w354 w418 _ _ _ w547 w553 w581 w603 w620 w643]
      tunnel: w260 -> [w265 w284 w359 w419 w488 w529 w539 w548 w557 w586 w599 w619 _]
      tunnel: [w263 errorcluster {"status"=FALSE, "code"=0, "source"=""} ("sortie d'erreur") w355 w422 w486 w527 w537 w548 w558 w582 w600 w618 w645] -> w255
      tunnel: [_ _ _ _ _ _ _ _ _ _ TRUE _ _] -> w262
      tunnel: w259 -> [_ _ _ _ _ _ _ _ w556 w585 w596 _ _]
      tunnel: w254 -> [_ _ _ _ w477 w530 w540 _ _ w560 _ _ _]
      tunnel: [w264 w281 w353 w423 w487 w528 w538 w547 w553 w581 w603 w617 w643] -> w253
      tunnel: [w273 w293 w362 w421 w485 w526 w536 w546 w552 w580 w595 w625 w642] -> w252
      tunnel: w251 -> [w273 _ w362 w421 w485 w526 w536 w546 w552 w580 w595 w625 w642]
      tunnel: [w272 w292 w360 w426 w480 w525 w535 w545 w551 w579 _ _ w641] -> w250
      tunnel: w249 -> [w272 w291 w361 w426 w480 w525 w535 w545 w551 w579 w591 w622 w641]
      tunnel: [w271 w290 w358 w420 w478 w523 w533 w543 w549 w577 w594 w624 w639] -> w248
      tunnel: w247 -> [w271 _ w358 w420 w478 w523 w533 w543 w549 w577 w594 w624 w639]
      tunnel: [w270 w289 w356 w425 w479 w524 w534 w544 w550 w578 _ _ w640] -> w246
      tunnel: w245 -> [w270 w288 w357 w425 w479 w524 w534 w544 w550 w578 w593 w623 w640]
      tunnel: w242 -> [_ _ _ _ _ _ _ _ _ _ w588 _ _]
      frame "Initialize" {
        n111 = local read "Type External"() -> (w267:enum16{"PS4 commander", "Other"})
        n112 = local read "Type Comm"() -> (w268:T28)
        n113 = case shown="\"External Commander\", Par défaut" w268 {
          tunnel: w267 -> [w275 _]
          frame "External Commander", Default {
            n114 = case shown="\"PS4 commander\", Par défaut" w275 {
              frame "PS4 commander", Default {
                n115 = local write "External_C"(enum32{"PS4", "OTHER"}."PS4" ("External_C")) -> ()
              }
              frame "Other" {
                n116 = local write "External_C"(enum32{"PS4", "OTHER"}."OTHER" ("External_C")) -> ()
              }
            }
            n117 = local write "Tab Control"(Onglet."External Commander" ("Tab Control")) -> ()
          }
          frame "Internal Commander" {
            n118 = local write "Tab Control"(Onglet."Internal Commander" ("Tab Control")) -> ()
          }
        }
        n119 = property on="External_C" class="Onglet (strict)"("Tabs Visible?"=FALSE ("Onglets visibles ?")) -> ()  [unwired: 2 in, 2 out]
        n120 = Flush Queue(queue=w266, error in (no error)=w265) -> (queue out=w264:refnum<queue>, error out=w263:errorcluster)  [unwired: 1 out]
      }
      frame "Open_Controller" {
        # "Initialize - All initialization work should take place in this message, since other loops can potentially enqueue messages that execute immediately after this one."
        n121 = local read "Type Comm"() -> (w293:T28)
        n122 = local read "Type External"() -> (w290:enum16{"PS4 commander", "Other"})
        n123 = Flush Queue(queue=w285, error in (no error)=w284) -> (queue out=w282:refnum<queue>, error out=w283:errorcluster)  [unwired: 1 out]
        n124 = case shown="\"External Commander\", Par défaut" w293 {
          tunnel: w282 -> [w303 w350]
          tunnel: w283 -> [w300 w349]
          tunnel: [w303 w350] -> w281
          tunnel: [w295 w349] -> w280
          tunnel: [w302 w348] -> w292
          tunnel: w291 -> [w301 w348]
          tunnel: w290 -> [w299 _]
          tunnel: [w298 w347] -> w289
          tunnel: w288 -> [w297 w347]
          tunnel: [w296 TRUE] -> w287
          frame "External Commander", Default {
            n125 = case shown="\"PS4 commander\", Par défaut" w299 {
              tunnel: [w311 w330] -> w295
              tunnel: [w312 w329] -> w302
              tunnel: w301 -> [w312 w328]
              tunnel: w300 -> [w307 w325]
              tunnel: [w309 w324] -> w298
              tunnel: w297 -> [w305 w324]
              tunnel: [w308 w323] -> w296
              frame "PS4 commander", Default {
                # "1."
                n126 = call <vilib>:"Close.vi"("Error In"=w307, "PS4 Controller Ref"=w305) -> ("Error Out"=w306:errorcluster)  [unwired: 9 in]
                n127 = while {
                  tunnel: w307 -> [w321]
                  tunnel: [w315] -> w311
                  shift-right: [w319] -> _
                  shift-left: 0 -> [w318]
                  tunnel: [w314] -> w309
                  tunnel: [w313] -> w308
                  tunnel: w306 -> [_]
                  stop <- w317 stop-if-true
                  n128 = call-poly <vilib>:"Open.vi"("Error In"=w321) -> ("Error Out"=w315:errorcluster, "PS4 Controller Ref"=w314:T32)  [unwired: 8 in, 1 out]
                  n129 = Increment(x=w318) -> (x+1=w319:i32)
                  n130 = Not(x=w315) -> (.not. x?=w316:bool)
                  n131 = Greater Or Equal?(x=w318, y=5) -> (x >= y?=w313:bool)
                  n132 = Or(x=w313, y=w316) -> (x .or. y?=w317:bool)
                  n133 = call "Non Manet2"("Enable"=w313) -> ()  [unwired: 9 in, 2 out]
                }
                n134 = local write "External_C"(enum32{"PS4", "OTHER"}."PS4" ("External_C")) -> ()
              }
              frame "Other" {
                n135 = call-poly <vilib>:"Close Input Device.vi"("error in (no error)"=w325, "device ID"=w328) -> ("error out"=w326:errorcluster)  [unwired: 8 in]
                n136 = while {
                  tunnel: [w340] -> w329
                  tunnel: w325 -> [w339]
                  tunnel: [w338] -> w330
                  tunnel: w326 -> [_]
                  shift-right: [w336] -> _
                  shift-left: 0 -> [w337]
                  tunnel: [w331] -> w323
                  stop <- w333 stop-if-true
                  # "Init Joystick"
                  n137 = call <vilib>:"Query Input Devices.vi"("error in (no error)"=w339) -> ("error out"=w344:errorcluster, "joystick info"=w341:T33)  [unwired: 7 in, 2 out]
                  n138 = Array Size(array=w341) -> (size(s)=w334:i32)
                  "Nuber of joysticks found:" <- w334
                  n139 = Index Array(array=w341, index="Joystick Number") -> (element=→"Joystick in Use":T21)
                  n140 = Increment(x=w337) -> (x+1=w336:i32)
                  n141 = call <vilib>:"Initialize Joystick.vi"("error in (no error)"=w344, "device index"="Joystick Number") -> ("error out"=w338:errorcluster, "device ID"=w340:refnum<k1>)  [unwired: 8 in]
                  n142 = Greater Or Equal?(x=w336, y=5) -> (x >= y?=w331:bool)
                  n143 = Not Equal To 0?(x=w334) -> (x != 0?=w332:bool)
                  n144 = Or(x=w331, y=w332) -> (x .or. y?=w333:bool)
                  n145 = call "Non Manet"("Enable"=w331) -> ()  [unwired: 9 in, 2 out]
                }
                n146 = local write "External_C"(enum32{"PS4", "OTHER"}."OTHER" ("External_C")) -> ()
              }
            }
            n147 = local write "Tab Control"(Onglet."External Commander" ("Tab Control")) -> ()
          }
          frame "Internal Commander" {
            n148 = local write "Tab Control"(Onglet."Internal Commander" ("Tab Control")) -> ()
          }
        }
        "error_OpenManette 2" <- w280
        n149 = Not(x=w287) -> (.not. x?=→"Init_Controller_OK":bool)
      }
      frame "Commander" {
        n150 = case shown="\"External Commander\", Par défaut" w362 {
          tunnel: w361 -> [w376 w416]
          tunnel: [w375 w416] -> w360
          tunnel: w359 -> [w374 w414]
          tunnel: [w373 w414] -> w352
          tunnel: w358 -> [w372 _]
          tunnel: w357 -> [w371 w415]
          tunnel: [w370 w415] -> w356
          frame "External Commander", Default {
            n151 = case shown="\"PS4 commander\", Par défaut" w372 {
              tunnel: w376 -> [w384 w397]
              tunnel: [w384 w396] -> w375
              tunnel: w374 -> [w381 w395]
              tunnel: [w380 w394] -> w373
              tunnel: w371 -> [w379 w386]
              tunnel: [w378 w386] -> w370
              frame "PS4 commander", Default {
                # "2."
                n152 = call <vilib>:"Read.vi"("Error In"=w381, "PS4 Controller Ref"=w379) -> ("Error Out"=w380:errorcluster, "All Axis"=w383:T16, "Buttons"=w382:T15, "PS4 Controller Ref"=w378:T32)  [unwired: 6 in]
                "PS4 Buttons" <- w382
                "PS4 All Axis" <- w383
                n153 = call <vilib>:"Button And Axis To Controller.vi"("All Axis"=w383, "Buttons"=w382) -> ("PS4 Controller"=→"PS4 Controller":T2)  [unwired: 5 in]
              }
              frame "Other" {
                n154 = call-poly <vilib>:"Acquire Input Data.vi"("device ID"=w397, "error in (no error)"=w395) -> ("device ID"=w396:refnum<k1>, "axis info"=→"axis info":T18, "button info"=w392:T34, "direction info"=→"direction info":T20, "error out"=w394:errorcluster)  [unwired: 13 in]
                n155 = Cluster To Array(cluster=w392) -> (array=w387:bool[])
                n156 = Array To Cluster(array=w387) -> (cluster=→"button":T35)
                n157 = local read "Tab_Ref"() -> (w385:refnum<vi>[])
                n158 = for {
                  tunnel: w387 -> [w398] mode=indexing
                  shift-right: [w400] -> w389
                  shift-left: "" -> [w401]
                  tunnel: w385 -> [w399] mode=indexing
                  i -> [w402]
                  n159 = Equal?(x=w398, y=TRUE) -> (x = y?=w403:bool)
                  n160 = case shown="Vrai" w403 {
                    tunnel: w402 -> [_ w413]
                    tunnel: w401 -> [w405 w407]
                    tunnel: [w405 w406] -> w400
                    frame False {
                    }
                    frame True {
                      # "Button is pressed"
                      n161 = Increment(x=w413) -> (x+1=w409:i32)
                      n162 = Number To Decimal String(number=w409) -> (decimal integer string=w411:string)  [unwired: 1 in]
                      n163 = Concatenate Strings("Button ", w411, " is pressed\n") -> (w408:string)
                      n164 = Concatenate Strings(w407, w408) -> (w406:string)
                    }
                  }
                  n165 = property class="Bool (strict)"(reference=w399, "Value"=w398) -> ()  [unwired: 1 in, 2 out]
                }
                "Txt Display" <- w389
              }
            }
          }
          frame "Internal Commander" {
          }
        }
        n166 = case shown="Pas d'erreur" w352 {
          selector: w352 -> [w366 w368]
          tunnel: [w365 _] -> w355
          tunnel: w354 -> [w364 w369]
          tunnel: [w363 w369] -> w353
          frame No Error {
            n167 = call-poly "Enqueue Message.vi"("error in (no error)"=w366, "Message"="MJ", "Message Queue"=w364) -> ("error out"=w365:errorcluster, "dup Message Queue"=w363:refnum<queue>)  [unwired: 7 in]
          }
          frame Error {
            "error_Controller" <- w368
          }
        }
        n168 = Not(x=w352) -> (.not. x?=→"Controller_OK":bool)
      }
      frame "MJ" {
        n169 = case shown="\"External Commander\", Par défaut" w421 {
          tunnel: w420 -> [w429 _]
          tunnel: w419 -> [w427 w469]
          tunnel: [w428 w469] -> w417
          frame "External Commander", Default {
            n170 = case shown="\"PS4 commander\", Par défaut" w429 {
              tunnel: [w459 w463] -> w428
              tunnel: w427 -> [w459 w463]
              frame "PS4 commander", Default {
                n171 = local read "PS4 Buttons"() -> (w448:T15)
                n172 = local read "PS4 All Axis"() -> (w441:T16)
                n173 = local read "PS4 All Axis"() -> (w451:T16)
                n174 = Unbundle By Name(w448) -> ("Playstation Button"=w432:bool, "Circle"=w447:bool, "Triangle"=w446:bool, "Square"=w445:bool, "L1"=w443:bool, "R1"=w442:bool)
                n175 = Unbundle By Name(w441) -> ("D-Pad"=w440:T17)
                n176 = Unbundle By Name(w451) -> ("Left Thumbstick.X Axis"=w450:i32, "Left Thumbstick.Y Axis"=w452:i32, "Right Thumbstick.X Axis"=w453:i32, "Right Thumbstick.Y Axis"=w454:i32)
                n177 = case shown="\"Up\"" w440 {
                  tunnel: [_ 2 _ 1 _ _ _ 4 _] -> w439
                  frame "Idle", Default {
                  }
                  frame "Up" {
                  }
                  frame "Up / Right" {
                  }
                  frame "Right" {
                  }
                  frame "Down / Right" {
                  }
                  frame "Down" {
                  }
                  frame "Down / Left" {
                  }
                  frame "Left" {
                  }
                  frame "Up / Left" {
                  }
                }
                n178 = control-ref of="Stop_Hexap"() -> (w430:refnum<vi>)
                n179 = control-ref of="Start_Hexap"() -> (w431:refnum<vi>)
                n180 = Number To Boolean Array(number=w439) -> (Boolean array=w438:bool[])
                n181 = Array To Cluster(array=w438) -> (cluster=w437:T36)
                n182 = Unbundle By Name(w437) -> ("Boolean array[0]"=w436:bool, "Boolean array[1]"=w435:bool, "Boolean array[2]"=w434:bool)
                n183 = local read "Hexap_ON"() -> (w433:bool)
                n184 = call "HexpSS(sous-VI).vi"("Hexap_ON"=w433, "Playstation Button"=w432, "Stop_Hexap"=w430, "Start_Hexap"=w431) -> ()  [unwired: 8 in]
                n185 = call "Convert(SubVI).vi"("Left Thumbstick.X Axis"=w450) -> ("Numeric"=w455:u8)
                n186 = call "Convert(SubVI).vi"("Left Thumbstick.X Axis"=w452) -> ("Numeric"=w456:u8)
                n187 = call "Convert(SubVI).vi"("Left Thumbstick.X Axis"=w453) -> ("Numeric"=w457:u8)
                n188 = call "Convert(SubVI).vi"("Left Thumbstick.X Axis"=w454) -> ("Numeric"=w458:u8)
                n189 = local write "Left joystick Horizontal"(w455) -> ()
                n190 = local write "Left joystick Vertical"(w456) -> ()
                n191 = local write "Right joystick Horizontal"(w457) -> ()
                n192 = local write "Right  joystick Vertical"(w458) -> ()
                n193 = local read "Button"() -> (w449:T22)
                n194 = Bundle By Name(cluster=w449, "R1"=w447, "R2"=w446, "R3"=w445, "LT"=w443, "RT"=w442, "L4"=w436, "L5"=w435, "L6"=w434) -> (w444:T22)
                n195 = local write "Button"(w444) -> ()
              }
              frame "Other" {
                (unwired) FALSE ("Playstation Button")
              }
            }
          }
          frame "Internal Commander" {
            (unwired) FALSE ("Playstation Button")
            n196 = local write "Left joystick Horizontal"("Left joystick Horizontal 2") -> ()
            n197 = local write "Left joystick Vertical"("Left joystick Vertical 2") -> ()
            n198 = local write "Right joystick Horizontal"("Right joystick Horizontal 2") -> ()
            n199 = local write "Right  joystick Vertical"("Right  joystick Vertical 2") -> ()
            n200 = local write "Button"("Button 2") -> ()
          }
        }
        n201 = call-poly "Enqueue Message.vi"("error in (no error)"=w417, "Message"="New_Data_To_Send", "Message Queue"=w418) -> ("error out"=w422:errorcluster, "dup Message Queue"=w423:refnum<queue>)  [unwired: 7 in]
      }
      frame "New_Data_To_Send" {
        n202 = for {
          N: 8 -> [_]
          shift-right: [w501] -> w474
          shift-left: u8[] [] -> [w499]
          i -> [w503]
          n203 = case shown="5" w503 {
            tunnel: [u8 255 w506 w508 w510 w512 w514 u8 0 ("Right joystick Horizontal") u8 255] -> w502
            tunnel: [w504 w507 w509 w511 w513 w518 w520 w521] -> w500
            tunnel: w499 -> [w504 w507 w509 w511 w513 w518 w520 w521]
            frame 0, Default {
            }
            frame 1 {
              n204 = local read "Left joystick Vertical"() -> (w506:u8)
            }
            frame 2 {
              n205 = local read "Left joystick Horizontal"() -> (w508:u8)
            }
            frame 3 {
              n206 = local read "Right  joystick Vertical"() -> (w510:u8)
            }
            frame 4 {
              n207 = local read "Right joystick Horizontal"() -> (w512:u8)
            }
            frame 5 {
              n208 = local read "Button"() -> (w515:T22)
              n209 = Cluster To Array(cluster=w515) -> (array=w516:bool[])
              n210 = Boolean Array To Number(Boolean array=w516) -> (number=w517:u32)
              n211 = To Unsigned Byte Integer(number=w517) -> (unsigned 8bit integer=w514:u8)
            }
            frame 6 {
            }
            frame 7 {
            }
          }
          n212 = Build Array (concatenate)(w500, w502) -> (w501:u8[])
        }
        "Array" <- w474
        n213 = Byte Array To String(unsigned byte array=w474) -> (string=w472:string)
        n214 = Concatenate Strings(w472, "\r\n") -> (w473:string)
        n215 = String To Byte Array(string=w472) -> (unsigned byte array=→"Array 2":u8[])
        n216 = Bundle By Name(cluster=T31 {"Data"="", "COM"=""}, "Data"=w473) -> (w483:T31)
        n217 = Unbundle By Name(w477) -> ("UI"=w476:refnum<queue>)
        n218 = local read "Init_COM_OK"() -> (w475:bool)
        n219 = case shown="Vrai" w475 {
          tunnel: w488 -> [w489 w498]
          tunnel: w476 -> [w490 w497]
          tunnel: [w490 w496] -> w487
          tunnel: [w489 w495] -> w486
          tunnel: w483 -> [_ w493]
          frame False {
          }
          frame True {
            (unwired) "Reciev_Data" ("Message")
            n220 = To Variant(anything=w493) -> (Variant=w494:variant)
            n221 = call-poly "Enqueue Message.vi"("Priority Message? (F)"=TRUE, "error in (no error)"=w498, "Message Data"=w494, "Message"="Send_Data", "Message Queue"=w497) -> ("error out"=w495:errorcluster, "dup Message Queue"=w496:refnum<queue>)  [unwired: 5 in]
          }
        }
      }
      frame "Open_Visu" {
        n222 = Unbundle By Name(w530) -> ("UI 3"=w531:refnum<queue>)
        n223 = call-poly "Enqueue Message.vi"("error in (no error)"=w529, "Message"="Open_Visu", "Message Queue"=w531) -> ("error out"=w527:errorcluster, "dup Message Queue"=w528:refnum<queue>)  [unwired: 7 in]
      }
      frame "Visu_Data" {
        n224 = Unbundle By Name(w540) -> ("UI 3"=w541:refnum<queue>)
        n225 = call-poly "Enqueue Message.vi"("error in (no error)"=w539, "Message"="Respond_Visu_Data", "Message Queue"=w541) -> ("error out"=w537:errorcluster, "dup Message Queue"=w538:refnum<queue>)  [unwired: 7 in]
      }
      frame "Modif_Visu_Data" {
      }
      frame "Update Display" {
        # "Update Display - Convert the message data to a string to display in the Data Display indicator."
        n226 = Variant To Data(error in=w557, type="", Variant=w556) -> (error out=w554:errorcluster)  [unwired: 1 out]
        n227 = Merge Errors(w554) -> (w558:errorcluster)
      }
      frame "Error" {
        w572 = FALSE
        # "Error - Display an error dialog. This message is sent by the \"Error Handler\" VIs at the end of other loops in this application."
        n228 = Variant To Data(error in=w586, type=errorcluster {"status"=FALSE, "code"=0, "source"=""} ("error constant"), Variant=w585) -> (data=w583:errorcluster)  [unwired: 1 out]
        n229 = call <vilib>:"Simple Error Handler.vi"("error in (no error)"=w583) -> ()  [unwired: 4 in, 5 out]
        n230 = Unbundle By Name(w560) -> ("UI 3"=w562:refnum<queue>, "UI 2"=w566:refnum<queue>, "UI"=w569:refnum<queue>)
        n231 = call-poly "Enqueue Message.vi"("Priority Message? (F)"=TRUE, "Message"="Close_Com", "Message Queue"=w569) -> ("error out"=w565:errorcluster)  [unwired: 7 in, 1 out]
        n232 = property on="Stop COM" class="Bool (strict)"("Visible"=w572) -> (error out=w574:errorcluster)  [unwired: 2 in, 1 out]
        n233 = Not(x=w572) -> (.not. x?=w573:bool)
        n234 = property on="Start COM" class="Bool (strict)"(error in=w574, "Visible"=w573) -> ()  [unwired: 1 in, 2 out]
        n235 = call-poly "Enqueue Message.vi"("Priority Message? (F)"=TRUE, "error in (no error)"=w565, "Message"="Close_Contoller", "Message Queue"=w566) -> ("error out"=w561:errorcluster)  [unwired: 6 in, 1 out]
        n236 = local write "Start/Stop COM"(FALSE ("Start/Stop COM")) -> ()
        n237 = local write "Stop COM"(FALSE ("Stop COM")) -> ()
        n238 = call-poly "Enqueue Message.vi"("Priority Message? (F)"=TRUE, "error in (no error)"=w561, "Message"="Close_SSH", "Message Queue"=w562) -> ("error out"=w559:errorcluster)  [unwired: 6 in, 1 out]
        n239 = Merge Errors(w559) -> (w582:errorcluster)
      }
      frame "Exit" {
        # "Stop the VI"
        # "Release the message queue reference"
        # "Exit - Exit the application."
        n240 = Variant To Data(type=errorcluster {"status"=FALSE, "code"=0, "source"=""} ("error constant"), Variant=w596) -> (data=w597:errorcluster)  [unwired: 1 in, 1 out]
        n241 = call <vilib>:"Simple Error Handler.vi"("error in (no error)"=w597) -> ()  [unwired: 4 in, 5 out]
        n242 = local read "Init_Controller_OK"() -> (w590:bool)
        n243 = case shown="\"External Commander\", Par défaut" w595 {
          tunnel: w594 -> [w608 _]
          tunnel: w593 -> [w607 _]
          tunnel: [w606 _] -> w592
          tunnel: w591 -> [w605 _]
          tunnel: w590 -> [w604 _]
          frame "External Commander", Default {
            n244 = case shown="Vrai" w604 {
              tunnel: w608 -> [_ w612]
              tunnel: w607 -> [_ w611]
              tunnel: [_ w610] -> w606
              tunnel: w605 -> [_ w609]
              frame False {
              }
              frame True {
                n245 = case shown="\"PS4 commander\", Par défaut" w612 {
                  tunnel: w611 -> [w614 _]
                  tunnel: [w613 w615] -> w610
                  tunnel: w609 -> [_ w616]
                  frame "PS4 commander", Default {
                    n246 = call <vilib>:"Close.vi"("PS4 Controller Ref"=w614) -> ("Error Out"=w613:errorcluster)  [unwired: 10 in]
                  }
                  frame "Other" {
                    n247 = call-poly <vilib>:"Close Input Device.vi"("device ID"=w616) -> ("error out"=w615:errorcluster)  [unwired: 9 in]
                  }
                }
              }
            }
          }
          frame "Internal Commander" {
          }
        }
        n248 = call "Fire User Event - Stop.vi"("User Event - Stop"=w588) -> ("error out"=w587:errorcluster)  [unwired: 10 in]
        n249 = Release Queue(queue=w603, error in (no error)=w599) -> (error out=w601:errorcluster)  [unwired: 1 in, 2 out]
        n250 = property on="External_C" class="Onglet (strict)"("Tabs Visible?"=TRUE ("Onglets visibles ?")) -> ()  [unwired: 2 in, 2 out]
        n251 = Merge Errors(w587, w592, w601) -> (w600:errorcluster)
      }
      frame "Close_Contoller" {
        # "Exit - Exit the application."
        n252 = local read "Init_Controller_OK"() -> (w621:bool)
        n253 = case shown="\"External Commander\", Par défaut" w625 {
          tunnel: w624 -> [w630 _]
          tunnel: w623 -> [w629 _]
          tunnel: [w628 _] -> _
          tunnel: w622 -> [w627 _]
          tunnel: w621 -> [w626 _]
          frame "External Commander", Default {
            n254 = case shown="Vrai" w626 {
              tunnel: w630 -> [_ w634]
              tunnel: w629 -> [_ w633]
              tunnel: [_ w632] -> w628
              tunnel: w627 -> [_ w631]
              frame False {
              }
              frame True {
                n255 = case shown="\"PS4 commander\", Par défaut" w634 {
                  tunnel: w633 -> [w636 _]
                  tunnel: [w635 w637] -> w632
                  tunnel: w631 -> [_ w638]
                  frame "PS4 commander", Default {
                    n256 = call <vilib>:"Close.vi"("PS4 Controller Ref"=w636) -> ("Error Out"=w635:errorcluster)  [unwired: 10 in]
                  }
                  frame "Other" {
                    n257 = call-poly <vilib>:"Close Input Device.vi"("device ID"=w638) -> ("error out"=w637:errorcluster)  [unwired: 9 in]
                  }
                }
              }
            }
          }
          frame "Internal Commander" {
          }
        }
        n258 = Flush Queue(queue=w620, error in (no error)=w619) -> (queue out=w617:refnum<queue>, error out=w618:errorcluster)  [unwired: 1 out]
      }
      frame Default {
        # "'Default' case only runs if there is a message that isn't defined in any of the other cases.  Output a programming error."
        n259 = xnode "Error Ring"("paramètre 0"=w644) -> ("sortie d'erreur"=w645:errorcluster)
      }
    }
    n260 = call "Error Handler - Message Handling Loop.vi"("error in (no error)"=w255, "Message Queue"=w253) -> ("dup error in"=w256:errorcluster)  [unwired: 8 in, 1 out]
  }
  n261 = while {
    tunnel: w21 -> [w663]
    shift-right: [w669] -> _
    shift-left: T29 {"Boolean <Replace Me>"=FALSE, "String <Replace Me>"="", "Numeric <Replace Me>"=0.0, "Do Something Ref"=refnum, "Do Something Else Ref"=refnum, "Data Display Ref"=refnum, "Exit Button Ref"=refnum} ("Data Cluster") -> [w670]
    tunnel: w1 -> [w667]
    tunnel: w4 -> [w666]
    tunnel: [w661] -> w22
    tunnel: w10 -> [w659]
    shift-right: [w657] -> _
    shift-left: _ -> [w656]
    shift-right: [w653] -> _
    shift-left: FALSE -> [w654]
    stop <- w668 stop-if-true
    # "USB/WIFI"
    n262 = call "Dequeue Message.vi"("error in (no error)"=w666, "Message Queue"=w663) -> ("error out"=w665:errorcluster, "Message Data"=w664:variant, "Message"=w655:string, "dup Message Queue"=w662:refnum<queue>)  [unwired: 6 in]
    "Chaîne_USB/WIFI" <- w655
    n263 = case "Message Cases" shown="\"Send_Data\"" w655 {
      selector: w655 -> [_ _ _ _ _ _ _ _ _ w961]
      tunnel: w662 -> [w681 w696 w769 w786 w824 w882 w900 w921 w952 w960]
      tunnel: w665 -> [w682 w698 w771 w785 w823 w884 w899 w936 w942 _]
      tunnel: [w678 w692 w766 w784 w827 w878 w904 w931 w948 w962] -> w660
      tunnel: w670 -> [w689 w699 w775 w787 w828 w885 w905 w935 w951 w963]
      tunnel: [w689 w699 w775 w787 w828 w885 w905 w935 w951 w963] -> w669
      tunnel: [_ _ _ _ _ _ _ _ TRUE _] -> w668
      tunnel: w664 -> [_ _ _ _ w821 _ _ w934 w943 _]
      tunnel: w667 -> [_ _ _ _ _ _ _ _ w947 _]
      tunnel: w656 -> [_ w697 w765 w783 w826 w883 w896 w930 w941 w959]
      tunnel: w659 -> [_ _ _ _ _ _ w898 w922 _ _]
      tunnel: [w679 w691 w768 w786 w825 w877 w895 w921 w952 w960] -> w658
      tunnel: ["Type Connexion" w697 w765 w783 w826 w881 w896 w930 w941 w959] -> w657
      frame "Initialize" {
        w674 = FALSE
        w684 = FALSE
        # "Initialize - All initialization work should take place in this message, since other loops can potentially enqueue messages that execute immediately after this one."
        n264 = property on="Stop COM" class="Bool (strict)"(error in=w682, "Visible"=w684) -> (error out=w683:errorcluster)  [unwired: 1 in, 1 out]
        n265 = Not(x=w684) -> (.not. x?=w685:bool)
        n266 = local write "Chaîne"("" ("Receiv")) -> ()
        n267 = property on="Tab Control" class="Onglet (strict)"("Tabs Visible?"=FALSE ("Onglets visibles ?")) -> ()  [unwired: 2 in, 2 out]
        n268 = local write "Output"("") -> ()
        n269 = local write "COM_OK"(TRUE ("COM_OK")) -> ()
        n270 = local write "Start/Stop COM"(FALSE ("Start/Stop COM")) -> ()
        n271 = local write "Hexap_ON"(FALSE ("Hexap_ON")) -> ()
        n272 = property on="Start COM" class="Bool (strict)"(error in=w683, "Visible"=w685) -> (error out=w680:errorcluster)  [unwired: 1 in, 1 out]
        n273 = property on="Stop_Hexap" class="Bool (strict)"("Visible"=w674) -> (error out=w673:errorcluster)  [unwired: 2 in, 1 out]
        n274 = Not(x=w674) -> (.not. x?=w675:bool)
        n275 = property on="Start_Hexap" class="Bool (strict)"(error in=w673, "Visible"=w675) -> ()  [unwired: 1 in, 2 out]
        n276 = Flush Queue(queue=w681, error in (no error)=w680) -> (queue out=w679:refnum<queue>, error out=w678:errorcluster)  [unwired: 1 out]
      }
      frame "Open_Com" {
        # "Initialize - All initialization work should take place in this message, since other loops can potentially enqueue messages that execute immediately after this one."
        n277 = case shown="\"Connexion WIFI\"" w697 {
          tunnel: [w707 w728] -> w693
          tunnel: w698 -> [_ w735]
          tunnel: [w708 w729] -> w694
          tunnel: w696 -> [w708 w729]
          tunnel: [w706 w736] -> w690
          frame "Connexion USB", Default {
            # "Init USB"
            n278 = local read "USB"() -> (w709:T24)
            n279 = Unbundle By Name(w709) -> ("COM"=w715:refnum<visa-resource-name>)
            n280 = Equal?(x=refnum<visa-resource-name> refnum ("VISA resource name 2"), y=w715) -> (x = y?=w719:bool)
            n281 = call "Config_Com_USB.vi"("Enable"=w719, "USB"=w709) -> ("USB"=w717:T24, "OK"=w718:bool)  [unwired: 15 in, 1 out]
            n282 = Select(t=w717, s=w718, f=w709) -> (s? t:f=w701:T24)
            n283 = Unbundle By Name(w701) -> ("timeout (10sec)"=w700:u32, "COM"=w704:refnum<visa-resource-name>, "baud rate (9600)"=w714:u32, "data bits (8)"=w713:u16, "parity (0:none)"=w712:enum16{"None", "Odd", "Even", "Mark", "Space"}, "stop bits (10: 1 bit)"=w711:u16, "flow control (0:none)"=w710:u16)
            n284 = call-poly "VISA Configure Serial Port"("VISA resource name"=w704, "timeout (10sec)"=w700, "baud rate (9600)"=w714, "data bits (8)"=w713, "parity (0:none)"=w712, "stop bits (10: 1 bit)"=w711, "flow control (0:none)"=w710) -> ("VISA resource name out"=w705:refnum<visa-resource-name>, "error out"=w703:errorcluster)  [unwired: 7 in]
            n285 = VISA Open(error in (no error)=w703, VISA resource name=w705) -> (error out=w702:errorcluster)  [unwired: 3 in, 1 out]
            n286 = case shown="Erreur" w702 {
              selector: w702 -> [w720 w721]
              tunnel: [w720 _] -> w707
              frame No Error {
              }
              frame Error {
                "error_OpenUSB" <- w721
              }
            }
            n287 = local write "USB"(w701) -> ()
            n288 = Not(x=w702) -> (.not. x?=w706:bool)
          }
          frame "Connexion WIFI" {
            w726 = "" ("adresse")
            # "Init WIFI"
            n289 = local read "Connection Info."() -> (w727:T27)
            n290 = local read "TCP"() -> (w732:T23)
            n291 = Unbundle By Name(w732) -> ("adresse"=w734:string, "port"=w733:u16)
            n292 = Unbundle By Name(w727) -> ("Remote"=w722:string)
            n293 = Not Equal?(x=w726, y=w734) -> (x != y?=w723:bool)
            n294 = Not Equal?(x=w722, y=w726) -> (x != y?=w725:bool)
            n295 = Or(x=w725, y=w723) -> (x .or. y?=w724:bool)
            n296 = case shown="Vrai" w724 {
              tunnel: w735 -> [w743 w753]
              tunnel: [w744 w752] -> w728
              tunnel: w734 -> [_ w749]
              tunnel: w733 -> [w742 w751]
              tunnel: [w745 w750] -> w731
              tunnel: [w741 w748] -> w730
              tunnel: w723 -> [_ w747]
              tunnel: w722 -> [_ w746]
              frame False {
                n297 = call "Sans titre 3.vi"() -> ("Adresse IP 3"=w741:string)  [unwired: 19 in]
                n298 = TCP Open Connection(address=w741, remote port or service name=w742, error in (no error)=w743) -> (connection ID=w745:refnum<k5>, error out=w744:errorcluster)  [unwired: 2 in]
              }
              frame True {
                n299 = case shown="Vrai" w747 {
                  tunnel: w753 -> [w758 w763]
                  tunnel: [w757 w762] -> w752
                  tunnel: w751 -> [w756 w761]
                  tunnel: [w755 w760] -> w750
                  tunnel: w749 -> [_ w759]
                  tunnel: [w754 w759] -> w748
                  tunnel: w746 -> [w754 _]
                  frame False {
                    n300 = TCP Open Connection(address=w754, remote port or service name=w756, error in (no error)=w758) -> (connection ID=w755:refnum<k5>, error out=w757:errorcluster)  [unwired: 2 in]
                  }
                  frame True {
                    n301 = TCP Open Connection(address=w759, remote port or service name=w761, error in (no error)=w763) -> (connection ID=w760:refnum<k5>, error out=w762:errorcluster)  [unwired: 2 in]
                  }
                }
              }
            }
            n302 = case shown="Pas d'erreur" w728 {
              tunnel: w732 -> [w740 _]
              tunnel: w731 -> [w739 _]
              tunnel: w730 -> [w737 _]
              frame No Error {
                n303 = Bundle By Name(cluster=w740, "adresse"=w737, "connection ID"=w739) -> (w738:T23)
                n304 = local write "TCP"(w738) -> ()
              }
              frame Error {
              }
            }
            n305 = Not(x=w728) -> (.not. x?=w736:bool)
          }
        }
        "Init_COM_OK" <- w690
        n306 = call "NoCom(sous-VI).vi"("entrée d'erreur (pas d'erreur)"=w693, "Message Queue"=w694) -> ("error out"=w692:errorcluster, "dup Message Queue"=w691:refnum<queue>)  [unwired: 8 in]
        n307 = Not(x=w690) -> (.not. x?=w695:bool)
        n308 = call "Com"("Enable"=w695) -> ()  [unwired: 9 in, 2 out]
      }
      frame "NewCOM" {
        n309 = Flush Queue(queue=w769, error in (no error)=w771) -> (queue out=w770:refnum<queue>, error out=w767:errorcluster)  [unwired: 1 out]
        n310 = local read "Start/Stop COM"() -> (w764:bool)
        n311 = call-poly "Enqueue Message.vi"("error in (no error)"=w767, "Message"="Close_Com", "Message Queue"=w770) -> ("error out"=w772:errorcluster, "dup Message Queue"=w773:refnum<queue>)  [unwired: 7 in]
        n312 = case shown="Vrai" w764 {
          tunnel: w773 -> [w776 w782]
          tunnel: w772 -> [w777 w781]
          tunnel: [w776 w779] -> w768
          tunnel: [w777 w778] -> w766
          frame False {
          }
          frame True {
            n313 = call-poly "Enqueue Message.vi"("error in (no error)"=w781, "Message"="Open_Com", "Message Queue"=w782) -> ("error out"=w778:errorcluster, "dup Message Queue"=w779:refnum<queue>)  [unwired: 7 in]
          }
        }
      }
      frame "Read_Data" {
        n314 = case shown="\"Connexion WIFI\"" w783 {
          tunnel: w785 -> [w790 w809]
          tunnel: [w788 w808] -> w784
          frame "Connexion USB", Default {
            n315 = local read "USB"() -> (w794:T24)
            n316 = Unbundle By Name(w794) -> ("COM"=w789:refnum<visa-resource-name>)
            n317 = case shown="Vrai" TRUE {
              tunnel: [errorcluster {"status"=TRUE, "code"=1000, "source"="Brandon"} ("error out") w797] -> w793
              tunnel: ["" ("read buffer") w798] -> w792
              tunnel: w790 -> [_ w800]
              tunnel: w789 -> [_ w799]
              frame False {
              }
              frame True {
                n318 = VISA Read(VISA resource name=w799, byte count=u32 1, error in (no error)=w800) -> (read buffer=w798:string, error out=w797:errorcluster)  [unwired: 2 out]
                n319 = local write "error_"(w797) -> ()
              }
            }
            n320 = case shown="Pas d'erreur" w793 {
              selector: w793 -> [w804 _]
              tunnel: w792 -> [w805 _]
              tunnel: [w804 _] -> w788
              frame No Error {
                n321 = local read "Chaîne"() -> (w803:string)
                n322 = Concatenate Strings(w803, w805) -> (w802:string)
                n323 = local write "Chaîne"(w802) -> ()
              }
              frame Error {
              }
            }
          }
          frame "Connexion WIFI" {
            n324 = local read "TCP"() -> (w811:T23)
            n325 = Unbundle By Name(w811) -> ("connection ID"=w810:refnum<k5>, "timeout ms"=w812:i32)
            n326 = TCP Read(connection ID=w810, error in (no error)=w809, 9:w812) -> (data out=w807:string, error out=w806:errorcluster)  [unwired: 2 in, 1 out]
            n327 = local write "error_"(w806) -> ()
            n328 = case shown="Pas d'erreur" w806 {
              selector: w806 -> [w815 _]
              tunnel: w807 -> [w817 _]
              tunnel: [w815 _] -> w808
              frame No Error {
                n329 = local read "Chaîne"() -> (w814:string)
                n330 = Concatenate Strings(w814, "\r\n", w817) -> (w813:string)
                n331 = local write "Chaîne"(w813) -> ()
              }
              frame Error {
              }
            }
          }
        }
      }
      frame "Send_Data" {
        n332 = Variant To Data(error in=w823, type=T31 {"Data"="", "COM"=""}, Variant=w821) -> (data=w819:T31, error out=w822:errorcluster)
        n333 = case shown="\"Connexion WIFI\"" w826 {
          tunnel: [w835 w863] -> w827
          tunnel: w822 -> [w838 w863]
          tunnel: [w843 w872] -> w825
          tunnel: w824 -> [w843 w872]
          tunnel: w819 -> [w842 w868]
          tunnel: [w839 w871] -> w818
          frame "Connexion USB", Default {
            # "USB"
            n334 = local read "USB"() -> (w830:T24)
            n335 = Unbundle By Name(w842) -> ("Data"=w841:string)
            n336 = Unbundle By Name(w830) -> ("COM"=w829:refnum<visa-resource-name>)
            n337 = case shown="Vrai" "Send" {
              tunnel: w841 -> [_ w849]
              tunnel: [w845 w848] -> w840
              tunnel: w838 -> [w845 w847]
              tunnel: w829 -> [w844 w846]
              tunnel: [w844 w846] -> w831
              frame False {
              }
              frame True {
                n338 = VISA Write(VISA resource name=w846, write buffer=w849, error in (no error)=w847) -> (error out=w848:errorcluster)  [unwired: 2 out]
              }
            }
            "error_Send_Data" <- w840
            n339 = property class="Instr"(reference=w831) -> ("Bytes at Port"=w833:u32)  [unwired: 1 in, 2 out]
            n340 = Greater Than 0?(x=w833) -> (x > 0?=w834:bool)
            n341 = case shown="Vrai" w834 {
              tunnel: w838 -> [_ w856]
              tunnel: w831 -> [_ w855]
              tunnel: [errorcluster {"status"=TRUE, "code"=1000, "source"="Brandon"} ("error out") w852] -> w837
              tunnel: ["" ("read buffer") w853] -> w836
              tunnel: w833 -> [_ w854]
              frame False {
              }
              frame True {
                n342 = VISA Read(VISA resource name=w855, byte count=w854, error in (no error)=w856) -> (read buffer=w853:string, error out=w852:errorcluster)  [unwired: 2 out]
                n343 = local write "error_"(w852) -> ()
              }
            }
            n344 = case shown="Pas d'erreur" w837 {
              selector: w837 -> [w859 _]
              tunnel: w836 -> [w860 _]
              tunnel: [w859 _] -> w835
              frame No Error {
                n345 = local read "Chaîne"() -> (w858:string)
                n346 = Concatenate Strings(w858, w860) -> (w857:string)
                n347 = local write "Chaîne"(w857) -> ()
              }
              frame Error {
              }
            }
            n348 = Not(x=w840) -> (.not. x?=w839:bool)
          }
          frame "Connexion WIFI" {
            # "WIFI"
            n349 = local read "TCP"() -> (w865:T23)
            n350 = Unbundle By Name(w868) -> ("Data"=w867:string)
            n351 = Unbundle By Name(w865) -> ("connection ID"=w870:refnum<k5>)
            n352 = TCP Write(connection ID=w870, data in=w867, error in (no error)=w863) -> (connection ID out=w866:refnum<k5>, error out=w869:errorcluster)  [unwired: 2 out]
            n353 = local write "error_Send_Data"(w869) -> ()
            n354 = Unbundle By Name(w865) -> ("timeout ms"=w864:i32)
            n355 = TCP Read(connection ID=w866, error in (no error)=w863, 9:w864) -> (data out=w862:string, error out=w861:errorcluster)  [unwired: 2 in, 1 out]
            n356 = case shown="Pas d'erreur" w861 {
              tunnel: w862 -> [w876 _]
              frame No Error {
                n357 = local read "Chaîne"() -> (w874:string)
                n358 = Concatenate Strings(w874, "\r\n", w876) -> (w873:string)
                n359 = local write "Chaîne"(w873) -> ()
              }
              frame Error {
              }
            }
            n360 = local write "error_"(w861) -> ()
            n361 = Not(x=w863) -> (.not. x?=w871:bool)
          }
        }
        "COM_OK" <- w818
      }
      frame "Close_Com" {
        n362 = case shown="\"Connexion USB\", Par défaut" w883 {
          tunnel: [w887 w892] -> w879
          tunnel: w884 -> [w887 w892]
          tunnel: [w889 w893] -> w880
          tunnel: w882 -> [w889 w893]
          frame "Connexion USB", Default {
            # "Close USB"
            n363 = local read "USB"() -> (w886:T24)
            n364 = Unbundle By Name(w886) -> ("COM"=w888:refnum<visa-resource-name>)
            n365 = VISA Close(VISA resource name=w888, error in (no error)=w887) -> ()  [unwired: 1 out]
          }
          frame "Connexion WIFI" {
            # "Close WIFI"
            n366 = local read "TCP"() -> (w891:T23)
            n367 = Unbundle By Name(w891) -> ("connection ID"=w890:refnum<k5>)
            n368 = TCP Close Connection(connection ID=w890, error in (no error)=w892) -> ()  [unwired: 1 in, 2 out]
          }
        }
        n369 = local read "Type Connexion"() -> (w881:enum16{"Connexion USB", "Connexion WIFI"})
        n370 = Flush Queue(queue=w880, error in (no error)=w879) -> (queue out=w877:refnum<queue>, error out=w878:errorcluster)  [unwired: 1 out]
      }
      frame "Confirm Quit" {
        # "Confirm Quit - Message that can confirm whether or not the user wants to exit the application."
        n371 = call-poly "Enqueue Message.vi"("Priority Message? (F)"=TRUE, "error in (no error)"=w899, "Message"="Close_Com", "Message Queue"=w900) -> ("error out"=w894:errorcluster)  [unwired: 6 in, 1 out]
        n372 = Cluster To Array(cluster=w898) -> (array=w897:refnum<queue>[])
        n373 = for {
          shift-right: [w910] -> w903
          shift-left: w894 -> [w908]
          tunnel: w897 -> [w907] mode=indexing
          tunnel: [w906] -> w895
          # "All Exit"
          n374 = call-poly "Enqueue Message.vi"("error in (no error)"=w908, "Message"="Exit", "Message Queue"=w907) -> ("error out"=w910:errorcluster, "dup Message Queue"=w906:refnum<queue>)  [unwired: 7 in]
        }
        n375 = Merge Errors(w903) -> (w904:errorcluster)
      }
      frame "Error" {
        w920 = FALSE
        # "Error - Display an error dialog. This message is sent by the \"Error Handler\" VIs at the end of other loops in this application."
        n376 = Variant To Data(error in=w936, type=errorcluster {"status"=FALSE, "code"=0, "source"=""} ("error constant"), Variant=w934) -> (data=w932:errorcluster)  [unwired: 1 out]
        n377 = call <vilib>:"Simple Error Handler.vi"("error in (no error)"=w932) -> ()  [unwired: 4 in, 5 out]
        n378 = Unbundle By Name(w922) -> ("UI 3"=w913:refnum<queue>, "UI 2"=w924:refnum<queue>, "UI"=w927:refnum<queue>)
        n379 = call-poly "Enqueue Message.vi"("Priority Message? (F)"=TRUE, "Message"="Close_Com", "Message Queue"=w927) -> ("error out"=w923:errorcluster)  [unwired: 7 in, 1 out]
        n380 = property on="Stop COM" class="Bool (strict)"("Visible"=w920) -> (error out=w918:errorcluster)  [unwired: 2 in, 1 out]
        n381 = Not(x=w920) -> (.not. x?=w919:bool)
        n382 = call-poly "Enqueue Message.vi"("Priority Message? (F)"=TRUE, "error in (no error)"=w923, "Message"="Close_Contoller", "Message Queue"=w924) -> ("error out"=w912:errorcluster)  [unwired: 6 in, 1 out]
        n383 = property on="Start COM" class="Bool (strict)"(error in=w918, "Visible"=w919) -> ()  [unwired: 1 in, 2 out]
        n384 = local write "Start/Stop COM"(FALSE ("Start/Stop COM")) -> ()
        n385 = call-poly "Enqueue Message.vi"("Priority Message? (F)"=TRUE, "error in (no error)"=w912, "Message"="Close_SSH", "Message Queue"=w913) -> ("error out"=w911:errorcluster)  [unwired: 6 in, 1 out]
        n386 = local write "Stop COM"(FALSE ("Stop COM")) -> ()
        n387 = Merge Errors(w911) -> (w931:errorcluster)
      }
      frame "Exit" {
        w938 = FALSE
        # "Stop the VI"
        # "Release the message queue reference"
        # "Exit - Exit the application."
        n388 = Variant To Data(type=errorcluster {"status"=FALSE, "code"=0, "source"=""} ("error constant"), Variant=w943) -> (data=w944:errorcluster)  [unwired: 1 in, 1 out]
        n389 = call <vilib>:"Simple Error Handler.vi"("error in (no error)"=w944) -> ()  [unwired: 4 in, 5 out]
        n390 = case shown="\"Connexion WIFI\"" w941 {
          tunnel: w942 -> [w954 w956]
          frame "Connexion USB", Default {
            # "Close USB"
            n391 = local read "USB"() -> (w953:T24)
            n392 = Unbundle By Name(w953) -> ("COM"=w955:refnum<visa-resource-name>)
            n393 = VISA Close(VISA resource name=w955, error in (no error)=w954) -> ()  [unwired: 1 out]
          }
          frame "Connexion WIFI" {
            # "Close WIFI"
            n394 = local read "TCP"() -> (w958:T23)
            n395 = Unbundle By Name(w958) -> ("connection ID"=w957:refnum<k5>)
            n396 = TCP Close Connection(connection ID=w957, error in (no error)=w956) -> ()  [unwired: 1 in, 2 out]
          }
        }
        n397 = call "Fire User Event - Stop.vi"("User Event - Stop"=w947) -> ("error out"=w946:errorcluster)  [unwired: 10 in]
        n398 = Release Queue(queue=w952, error in (no error)=w942) -> (error out=w949:errorcluster)  [unwired: 1 in, 2 out]
        n399 = property on="Stop COM" class="Bool (strict)"("Visible"=w938) -> (error out=w937:errorcluster)  [unwired: 2 in, 1 out]
        n400 = Not(x=w938) -> (.not. x?=w939:bool)
        n401 = property on="Start COM" class="Bool (strict)"(error in=w937, "Visible"=w939) -> ()  [unwired: 1 in, 2 out]
        n402 = Merge Errors(w946, w949) -> (w948:errorcluster)
        n403 = property on="Tab Control" class="Onglet (strict)"("Tabs Visible?"=TRUE ("Onglets visibles ?")) -> ()  [unwired: 2 in, 2 out]
      }
      frame Default {
        # "'Default' case only runs if there is a message that isn't defined in any of the other cases.  Output a programming error."
        n404 = xnode "Error Ring"("paramètre 0"=w961) -> ("sortie d'erreur"=w962:errorcluster)
      }
    }
    n405 = Not(x=w654) -> (.not. x?=w653:bool)
    "USB/WIFI" <- w653
    "StatCom" <- w653
    n406 = call "Error Handler - Message Handling Loop.vi"("error in (no error)"=w660, "Message Queue"=w658) -> ("dup error in"=w661:errorcluster)  [unwired: 8 in, 1 out]
  }
  n407 = while {
    shift-right: [w979] -> w17
    shift-left: w13 -> [w980]
    tunnel: [w975] -> w14
    tunnel: w10 -> [w974]
    shift-right: [w972] -> _
    shift-left: FALSE -> [w973]
    stop <- w977 stop-if-true
    # "Event Handling Loop"
    n408 = Not(x=w973) -> (.not. x?=w972:bool)
    "StatCom 2" <- w972
    n409 = event shown="[5] \"Preferences Button\": Valeur changée" {
      selector: w980 -> [_ _ _ _ _ _ _ _ _ _ _ _ _ _ _ _ _ _ _ _]
      dyn-events: [_ _ _ _ _ _ _ _ _ _ _ _ _ _ _ _ _ _ _ _] -> w979
      timeout: "Vitesse (ms)" -> [_ _ _ _ _ _ _ _ _ _ _ _ _ _ _ _ _ _ _ _]
      tunnel: [TRUE ("Discard?") _ _ _ _ _ _ _ _ _ _ _ _ _ _ _ _ _ _ TRUE ("Discard?")] -> w977
      tunnel: [w982 w992 _ _ _ _ w1014 w1024 w1060 w1068 w1070 w1085 w1088 w1102 _ _ _ _ w1160 _] -> w978
      tunnel: [w984 w993 _ _ _ _ w1015 w1025 w1059 w1067 w1071 w1084 w1087 w1103 _ _ _ _ w1161 w1174] -> w976
      tunnel: w974 -> [w983 w994 _ _ _ _ w1013 w1026 w1054 w1062 w1069 w1079 w1094 w1104 w1116 w1125 w1133 w1143 w1157 w1173]
      event Panel Close? {
        n410 = event-data() -> ()  [unwired: 1 in, 1 out]
        n411 = Cluster To Array(cluster=w983) -> (array=w985:refnum<queue>[])
        n412 = for {
          tunnel: [w990] -> w984
          tunnel: w985 -> [w989] mode=indexing
          tunnel: [w987] -> w982
          n413 = call-poly "Enqueue Message.vi"("Priority Message? (F)"=TRUE, "Message"="Exit", "Message Queue"=w989) -> ("error out"=w987:errorcluster, "dup Message Queue"=w990:refnum<queue>)  [unwired: 7 in]
        }
        n414 = event-data("Discard?"=TRUE) -> ()  [unwired: 1 in, 1 out]
      }
      event Application Instance Close {
        n415 = event-data() -> ()  [unwired: 1 in, 1 out]
        n416 = Cluster To Array(cluster=w994) -> (array=w995:refnum<queue>[])
        n417 = for {
          tunnel: [w999] -> w993
          tunnel: w995 -> [w998] mode=indexing
          tunnel: [w996] -> w992
          n418 = call-poly "Enqueue Message.vi"("Priority Message? (F)"=TRUE, "Message"="Exit", "Message Queue"=w998) -> ("error out"=w996:errorcluster, "dup Message Queue"=w999:refnum<queue>)  [unwired: 7 in]
        }
      }
      event "Home Button": Value Change {
        n419 = event-data() -> ()  [unwired: 1 in, 1 out]
        n420 = local read "Type Comm"() -> (w1002:T28)
        n421 = case shown="\"Internal Commander\"" w1002 {
          tunnel: [Onglet."External Commander" ("Tab Control") Onglet."Internal Commander" ("Tab Control")] -> w1001
          frame "External Commander", Default {
          }
          frame "Internal Commander" {
          }
        }
        n422 = local write "Tab Control"(w1001) -> ()
      }
      event "Settings Button": Value Change {
        n423 = event-data() -> ("NewVal"=w1005:bool)  [unwired: 1 in]
        n424 = case shown="Vrai" w1005 {
          frame False {
          }
          frame True {
            n425 = local write "Tab Control"(Onglet."Config Com" ("Tab Control")) -> ()
          }
        }
      }
      event "Putty": Value Change {
        n426 = event-data() -> ("NewVal"=w1007:bool)  [unwired: 1 in]
        n427 = case shown="Vrai" w1007 {
          frame False {
          }
          frame True {
            n428 = local write "Tab Control"(Onglet."SSH" ("Tab Control")) -> ()
            n429 = local write "Putty"(FALSE ("Putty")) -> ()
          }
        }
      }
      event "Preferences Button": Value Change {
        n430 = event-data() -> ("NewVal"=w1010:bool)  [unwired: 1 in]
        n431 = case shown="Vrai" w1010 {
          frame False {
          }
          frame True {
            n432 = local write "Tab Control"(T37."Debug" ("Tab Control")) -> ()
          }
        }
      }
      event "Search Button": Value Change {
        n433 = event-data() -> ("NewVal"=w1012:bool)  [unwired: 1 in]
        n434 = case shown="Vrai" w1012 {
          tunnel: [w1017 w1022] -> w1015
          tunnel: [_ w1021] -> w1014
          tunnel: w1013 -> [w1016 w1019]
          frame False {
            n435 = Unbundle By Name(w1016) -> ("UI 3"=w1017:refnum<queue>)
          }
          frame True {
            n436 = Unbundle By Name(w1019) -> ("UI 2"=w1018:refnum<queue>)
            n437 = call-poly "Enqueue Message.vi"("Message"="Open_Visu", "Message Queue"=w1018) -> ("error out"=w1021:errorcluster, "dup Message Queue"=w1022:refnum<queue>)  [unwired: 8 in]
          }
        }
      }
      event "R/W": Value Change {
        n438 = event-data() -> ("NewVal"=w1027:bool)  [unwired: 1 in]
        n439 = Unbundle By Name(w1026) -> ("UI 4"=w1023:refnum<queue>)
        n440 = disable-structure shown="Activé" {
          disable-tunnel: w1027 -> [w1031 w1050]
          disable-tunnel: [w1030 w1049] -> w1025
          disable-tunnel: [w1029 _] -> w1024
          disable-tunnel: w1023 -> [w1028 w1048]
          frame Disabled {
            n441 = case shown="Vrai" w1031 {
              tunnel: [w1035 w1043] -> w1030
              tunnel: [w1034 w1042] -> w1029
              tunnel: w1028 -> [w1033 w1041]
              frame True {
                n442 = local read "USB"() -> (w1037:T24)
                n443 = Unbundle By Name(w1037) -> ("COM"=w1036:refnum<visa-resource-name>)
                n444 = To Variant(anything=w1036) -> (Variant=w1038:variant)
                n445 = call-poly "Enqueue Message.vi"("Priority Message? (F)"=TRUE, "Message Data"=w1038, "Message"="Start_Read", "Message Queue"=w1033) -> ("error out"=w1034:errorcluster, "dup Message Queue"=w1035:refnum<queue>)  [unwired: 6 in]
              }
              frame False {
                n446 = local read "USB"() -> (w1045:T24)
                n447 = Unbundle By Name(w1045) -> ("COM"=w1044:refnum<visa-resource-name>)
                n448 = To Variant(anything=w1044) -> (Variant=w1046:variant)
                n449 = call-poly "Enqueue Message.vi"("Priority Message? (F)"=TRUE, "Message Data"=w1046, "Message"="Stop_Read", "Message Queue"=w1041) -> ("error out"=w1042:errorcluster, "dup Message Queue"=w1043:refnum<queue>)  [unwired: 6 in]
              }
            }
          }
          frame Enabled {
            n450 = case shown="Faux" w1050 {
              tunnel: [w1051 w1052] -> w1049
              tunnel: w1048 -> [w1051 w1052]
              frame False {
              }
              frame True {
              }
            }
          }
        }
      }
      event "Type Connexion": Value Change {
        n451 = event-data() -> ("NewVal"=w1058:enum16{"Connexion USB", "Connexion WIFI"})  [unwired: 1 in]
        n452 = Unbundle By Name(w1054) -> ("UI"=w1053:refnum<queue>)
        n453 = To Variant(anything=w1058) -> (Variant=w1056:variant)
        n454 = call-poly "Enqueue Message.vi"("Priority Message? (F)"=TRUE, "Message Data"=w1056, "Message"="NewCOM", "Message Queue"=w1053) -> ("error out"=w1060:errorcluster, "dup Message Queue"=w1059:refnum<queue>)  [unwired: 6 in]
      }
      event "Type Comm": Value Change {
        n455 = event-data() -> ("NewVal"=w1066:T28)  [unwired: 1 in]
        n456 = Unbundle By Name(w1062) -> ("UI 2"=w1061:refnum<queue>)
        n457 = To Variant(anything=w1066) -> (Variant=w1064:variant)
        n458 = call-poly "Enqueue Message.vi"("Priority Message? (F)"=TRUE, "Message Data"=w1064, "Message"="Initialize", "Message Queue"=w1061) -> ("error out"=w1068:errorcluster, "dup Message Queue"=w1067:refnum<queue>)  [unwired: 6 in]
      }
      event "Type External": Value Change {
        n459 = event-data() -> ("NewVal"=w1075:enum16{"PS4 commander", "Other"})  [unwired: 1 in]
        n460 = case shown="\"Other\"" w1075 {
          frame "PS4 commander", Default {
            n461 = local write "External_C"(enum32{"PS4", "OTHER"}."PS4" ("External_C")) -> ()
          }
          frame "Other" {
            n462 = local write "External_C"(enum32{"PS4", "OTHER"}."OTHER" ("External_C")) -> ()
          }
        }
        n463 = Unbundle By Name(w1069) -> ("UI 2"=w1072:refnum<queue>)
        n464 = call-poly "Enqueue Message.vi"("Priority Message? (F)"=TRUE, "Message"="Initialize", "Message Queue"=w1072) -> ("error out"=w1070:errorcluster, "dup Message Queue"=w1071:refnum<queue>)  [unwired: 7 in]
      }
      event "USB.COM": Value Change {
        n465 = event-data() -> ("NewVal"=w1083:refnum<visa-resource-name>)  [unwired: 1 in]
        n466 = Unbundle By Name(w1079) -> ("UI"=w1078:refnum<queue>)
        n467 = To Variant(anything=w1083) -> (Variant=w1081:variant)
        n468 = call-poly "Enqueue Message.vi"("Priority Message? (F)"=TRUE, "Message Data"=w1081, "Message"="NewCOM", "Message Queue"=w1078) -> ("error out"=w1085:errorcluster, "dup Message Queue"=w1084:refnum<queue>)  [unwired: 6 in]
      }
      event "Start COM": Value Change {
        w1099 = TRUE
        n469 = event-data() -> ()  [unwired: 1 in, 1 out]
        n470 = property on="Stop COM" class="Bool (strict)"("Visible"=w1099) -> (error out=w1098:errorcluster)  [unwired: 2 in, 1 out]
        n471 = Unbundle By Name(w1094) -> ("UI 2"=w1090:refnum<queue>, "UI"=w1093:refnum<queue>)
        n472 = Not(x=w1099) -> (.not. x?=w1100:bool)
        n473 = property on="Start COM" class="Bool (strict)"(error in=w1098, "Visible"=w1100) -> ()  [unwired: 1 in, 2 out]
        n474 = call-poly "Enqueue Message.vi"("Priority Message? (F)"=TRUE, "Message"="Open_Com", "Message Queue"=w1093) -> ("error out"=w1089:errorcluster)  [unwired: 7 in, 1 out]
        n475 = call-poly "Enqueue Message.vi"("Priority Message? (F)"=TRUE, "error in (no error)"=w1089, "Message"="Open_Controller", "Message Queue"=w1090) -> ("error out"=w1088:errorcluster, "dup Message Queue"=w1087:refnum<queue>)  [unwired: 6 in]
        n476 = local write "Start/Stop COM"(TRUE ("Start/Stop COM")) -> ()
        n477 = local write "Start COM"(FALSE ("Start COM")) -> ()
      }
      event "Stop COM": Value Change {
        w1113 = FALSE
        n478 = event-data() -> ()  [unwired: 1 in, 2 out]
        n479 = property on="Stop COM" class="Bool (strict)"("Visible"=w1113) -> ()  [unwired: 2 in, 2 out]
        n480 = Not(x=w1113) -> (.not. x?=w1114:bool)
        n481 = property on="Start COM" class="Bool (strict)"("Visible"=w1114) -> ()  [unwired: 2 in, 2 out]
        n482 = Unbundle By Name(w1104) -> ("UI 2"=w1106:refnum<queue>, "UI"=w1109:refnum<queue>)
        n483 = call-poly "Enqueue Message.vi"("Priority Message? (F)"=TRUE, "Message"="Close_Com", "Message Queue"=w1109) -> ("error out"=w1105:errorcluster)  [unwired: 7 in, 1 out]
        n484 = call-poly "Enqueue Message.vi"("Priority Message? (F)"=TRUE, "error in (no error)"=w1105, "Message"="Close_Contoller", "Message Queue"=w1106) -> ("error out"=w1102:errorcluster, "dup Message Queue"=w1103:refnum<queue>)  [unwired: 6 in]
        n485 = local write "Start/Stop COM"(FALSE ("Start/Stop COM")) -> ()
        n486 = local write "Stop COM"(FALSE ("Stop COM")) -> ()
      }
      event "Send_L": Value Change {
        n487 = event-data() -> ("NewVal"=w1115:bool)  [unwired: 1 in]
        n488 = case shown="Vrai" w1115 {
          tunnel: w1116 -> [_ w1118]
          frame False {
          }
          frame True {
            n489 = local read "Connected"() -> (w1117:bool)
            n490 = case shown="Vrai" w1117 {
              tunnel: w1118 -> [_ w1123]
              frame False {
              }
              frame True {
                n491 = Unbundle By Name(w1123) -> ("UI 3"=w1122:refnum<queue>)
                n492 = To Variant(anything="Commande") -> (Variant=w1121:variant)
                n493 = call-poly "Enqueue Message.vi"("Priority Message? (F)"=TRUE, "Message Data"=w1121, "Message"="Send_Com_SSH", "Message Queue"=w1122) -> ()  [unwired: 6 in, 2 out]
              }
            }
          }
        }
      }
      event "SSH_Connect": Value Change {
        n494 = event-data() -> ("NewVal"=w1126:bool)  [unwired: 1 in]
        n495 = case shown="Vrai" w1126 {
          tunnel: w1125 -> [_ w1128]
          frame False {
          }
          frame True {
            n496 = local read "Connected"() -> (w1127:bool)
            n497 = case shown="Faux" w1127 {
              tunnel: w1128 -> [w1130 _]
              frame False {
                n498 = Unbundle By Name(w1130) -> ("UI 3"=w1132:refnum<queue>)
                n499 = call-poly "Enqueue Message.vi"("Priority Message? (F)"=TRUE, "Message"="Open_SSH", "Message Queue"=w1132) -> ()  [unwired: 7 in, 2 out]
              }
              frame True {
              }
            }
          }
        }
      }
      event "Stop_Hexap": Value Change {
        n500 = event-data() -> ("NewVal"=w1134:bool)  [unwired: 1 in]
        n501 = case shown="Vrai" w1134 {
          tunnel: w1133 -> [_ w1138]
          frame False {
          }
          frame True {
            w1141 = FALSE
            n502 = Unbundle By Name(w1138) -> ("UI 3"=w1137:refnum<queue>)
            n503 = call-poly "Enqueue Message.vi"("Priority Message? (F)"=TRUE, "Message"="Stop_Hexap", "Message Queue"=w1137) -> ()  [unwired: 7 in, 2 out]
            n504 = local write "Stop_Hexap"(FALSE ("Stop_Hexap")) -> ()
            n505 = property on="Stop_Hexap" class="Bool (strict)"("Visible"=w1141) -> (error out=w1142:errorcluster)  [unwired: 2 in, 1 out]
            n506 = Not(x=w1141) -> (.not. x?=w1140:bool)
            n507 = property on="Start_Hexap" class="Bool (strict)"(error in=w1142, "Visible"=w1140) -> ()  [unwired: 1 in, 2 out]
          }
        }
      }
      event "Start_Hexap": Value Change {
        n508 = event-data() -> ("NewVal"=w1144:bool)  [unwired: 1 in]
        n509 = case shown="Vrai" w1144 {
          tunnel: w1143 -> [_ w1147]
          frame False {
          }
          frame True {
            w1151 = TRUE
            n510 = Unbundle By Name(w1147) -> ("UI 3"=w1149:refnum<queue>)
            n511 = call-poly "Enqueue Message.vi"("Priority Message? (F)"=TRUE, "Message"="Start_Hexap", "Message Queue"=w1149) -> ()  [unwired: 7 in, 2 out]
            n512 = local write "Start_Hexap"(FALSE ("Start_Hexap")) -> ()
            n513 = property on="Stop_Hexap" class="Bool (strict)"("Visible"=w1151) -> (error out=w1152:errorcluster)  [unwired: 2 in, 1 out]
            n514 = Not(x=w1151) -> (.not. x?=w1150:bool)
            n515 = property on="Start_Hexap" class="Bool (strict)"(error in=w1152, "Visible"=w1150) -> ()  [unwired: 1 in, 2 out]
          }
        }
      }
      event Timeout {
        n516 = event-data() -> ()  [unwired: 1 in, 2 out]
        n517 = local read "Connected"() -> (w1153:bool)
        n518 = local read "Hexap_ON"() -> (w1155:bool)
        n519 = Compound Arithmetic op=AND ("Opérateur arithmétique")(w1153, w1155) -> (w1154:bool)
        n520 = case shown="Vrai" w1154 {
          tunnel: w1157 -> [_ w1164]
          tunnel: [_ w1162] -> w1156
          frame False {
          }
          frame True {
            n521 = Unbundle By Name(w1164) -> ("UI 3"=w1163:refnum<queue>)
            n522 = call-poly "Enqueue Message.vi"("Message"="Read_Com_SSH", "Message Queue"=w1163) -> ("error out"=w1162:errorcluster)  [unwired: 8 in, 1 out]
          }
        }
        n523 = Unbundle By Name(w1157) -> ("UI 2"=w1159:refnum<queue>)
        n524 = local read "Start/Stop COM"() -> (w1158:bool)
        n525 = case shown="Vrai" w1158 {
          tunnel: [w1167 w1170] -> w1161
          tunnel: [w1166 w1169] -> w1160
          tunnel: w1159 -> [w1167 w1171]
          tunnel: w1156 -> [w1166 w1168]
          frame False {
          }
          frame True {
            n526 = call-poly "Enqueue Message.vi"("error in (no error)"=w1168, "Message"="Commander", "Message Queue"=w1171) -> ("error out"=w1169:errorcluster, "dup Message Queue"=w1170:refnum<queue>)  [unwired: 7 in]
          }
        }
      }
      event User Event {
        # "The Message Handling Loop processed an \"Exit\" message, which fired this event to stop the Event Handling Loop."
        n527 = event-data() -> ()  [unwired: 1 in, 1 out]
        n528 = Cluster To Array(cluster=w1173) -> (array=w1175:refnum<queue>[])
        n529 = for {
          tunnel: [w1179] -> w1174
          tunnel: w1175 -> [w1178] mode=indexing
          n530 = call-poly "Enqueue Message.vi"("Priority Message? (F)"=TRUE, "Message"="Exit", "Message Queue"=w1178) -> ("dup Message Queue"=w1179:refnum<queue>)  [unwired: 7 in, 1 out]
        }
      }
    }
    n531 = call "Error Handler - Event Handling Loop.vi"("error in (no error)"=w978, "Message Queue"=w976) -> ("dup error in"=w975:errorcluster)  [unwired: 8 in, 1 out]
  }
  n532 = Unregister For Events(event registration refnum=w17, error in=w14) -> (error out=w18:errorcluster)
  n533 = Merge Errors(w18, w22, w11, w9) -> (w19:errorcluster)
  n534 = call "Destroy User Event - Stop.vi"("error in (no error)"=w19, "User Event - Stop"=w1) -> ("error out"=w15:errorcluster)  [unwired: 9 in]
  n535 = global write "Global_1.vi" "Prev Boolean"(TRUE ("Prev Boolean")) -> ()
  n536 = disable-structure shown="RUN_TIME_ENGINE==True" {
    disable-tunnel: w15 -> [_ _]
    frame condition #0 (active) {
    }
    frame condition #1 {
      # "Call Quit LabVIEW if running as a built application."
      n537 = Quit LabVIEW() -> ()  [unwired: 1 in]
    }
  }
